vi "obsleftright.vi"(11 "update":bool=TRUE) -> ()   [LabVIEW 2015]
uses:
  G_SEN.vi
  <vilib>/Analysis/1siggen.llb/Ramp Pattern by Delta.vi
  G_ALL.vi
  <vilib>/Analysis/polynomials.llb/nth Derivative of Polynomial (DBL).vi
  <vilib>/Analysis/polynomials.llb/Scalar Polynomial Evaluation (DBL).vi
  <vilib>/Analysis/NI_AALPro.lvlib
  G_LCM.vi
  <vilib>/Analysis/NI_AALBase.lvlib
panel:
  out "x_car":dbl[](array[numeric])=[0.9, 0.9, -0.9, -0.9, 0.9]
  out "y_car":dbl[](array[numeric])=[0.0, 3.7, 3.7, 0.0, 0.0]
  out "y_ramp":dbl[](array[numeric])=[-1.0, -0.75, -0.5, -0.25, 0.0, 0.25, 0.5, 0.75, 1.0, 1.25, 1.5, 1.75, 2.0, 2.25, 2.5, 2.75, 3.0, 3.25, 3.5, 3.75, 4.0, 4.25, 4.5, 4.75, 5.0, 5.25, 5.5, 5.75, 6.0]
  out "rin":dbl[](array[numeric])=[-3.7555, -4.035824427641933, -4.343004633055794, -4.681538421297181, -5.056978730736188, -5.476262963548993, -5.94817384988562, -6.483997508991062, -7.098484710034956, -7.811291873800975, -8.649206492141174, -9.649704845388673, -10.866875707952016, -12.381774570932784, -14.321624936294773, -16.89815033646731, -20.49170207506112, -25.860884248621495, -34.76835875277913, -52.46351887551581, -104.73868975677755, -4879.314687241169, 109.5221450101935, 53.65969083607183, 35.30050875601431, 26.160648564205243, 20.683909481852254, 17.031933528233147, 14.42018130844496, 12.457468347457555, 10.92689587838567, 9.698514680927435, 8.689722854776836, 7.845501286784753, 7.127786761742499, 6.509406661367354, 5.970443364939505, 5.495963884688509, 5.074551847557845, 4.697329415527146, 4.357288430183145, 4.048822433014104, 3.767392532060661]
  out "rout":dbl[](array[numeric])=[-6.67484683344869, -6.909909315632319, -7.171227643977352, -7.463266061634917, -7.791543962127691, -8.162965313825287, -8.586279637191614, -9.072740199574223, -9.637065431692674, -10.298880108215295, -11.084940970316678, -12.032694671041764, -13.196201733859061, -14.656491052798271, -16.540761487505993, -19.06071420501164, -22.596680760750772, -27.907248474466925, -36.75506579877062, -54.389516276148846, -106.60291935538585, -4881.116089584579, 111.38361625333661, 55.58297677916027, 37.28455108962819, 28.204394482615516, 22.786315752840025, 19.19197020662005, 16.636835086002, 14.729745540190233, 13.253825059177073, 12.079148971161162, 11.1231418929198, 10.330812895090412, 9.66412833436853, 9.095946298432954, 8.60638077752387, 8.180531095636704, 7.807013712346161, 7.476983986466357, 7.183467186008942, 6.920890394517821, 6.684748282923211]
  out "r":dbl[](array[numeric])=[-4.6555, -4.935824427641934, -5.2430046330557945, -5.581538421297181, -5.956978730736188, -6.376262963548993, -6.848173849885621, -7.3839975089910626, -7.9984847100349565, -8.711291873800976, -9.549206492141174, -10.549704845388673, -11.766875707952016, -13.281774570932784, -15.221624936294774, -17.79815033646731, -21.39170207506112, -26.760884248621494, -35.66835875277913, -53.36351887551581, -105.63868975677755, -4880.214687241169, 110.4221450101935, 54.55969083607183, 36.20050875601431, 27.06064856420524, 21.583909481852253, 17.931933528233145, 15.32018130844496, 13.357468347457555, 11.82689587838567, 10.598514680927435, 9.589722854776836, 8.745501286784753, 8.0277867617425, 7.409406661367354, 6.870443364939505, 6.395963884688509, 5.974551847557845, 5.597329415527146, 5.257288430183145, 4.948822433014104, 4.667392532060661]
  out "theta":dbl[](array[numeric])=[-3.141592653589793, -3.1315926535897933, -3.121592653589793, -3.1115926535897933, -3.101592653589793, -3.0915926535897933, -3.081592653589793, -3.0715926535897933, -3.061592653589793, -3.0515926535897933, -3.041592653589793, -3.0315926535897932, -3.021592653589793, -3.0115926535897932, -3.001592653589793, -2.991592653589793, -2.981592653589793, -2.971592653589793, -2.961592653589793, -2.951592653589793, -2.941592653589793, -2.931592653589793, -2.921592653589793, -2.911592653589793, -2.901592653589793, -2.891592653589793, -2.8815926535897933, -2.871592653589793, -2.861592653589793, -2.851592653589793, -2.8415926535897933, -2.831592653589793, -2.8215926535897933, -2.811592653589793, -2.8015926535897933, -2.791592653589793, -2.7815926535897932, -2.771592653589793, -2.7615926535897932, -2.751592653589793, -2.741592653589793, -2.731592653589793, -2.721592653589793, -2.711592653589793, -2.701592653589793, -2.691592653589793, -2.681592653589793, -2.671592653589793, -2.661592653589793, -2.651592653589793, -2.641592653589793, -2.6315926535897933, -2.621592653589793, -2.611592653589793, -2.601592653589793, -2.5915926535897933, -2.581592653589793, -2.571592653589793, -2.561592653589793, -2.5515926535897933, -2.541592653589793, -2.5315926535897932, -2.521592653589793, -2.5115926535897932, -2.501592653589793, -2.491592653589793, -2.481592653589793, -2.471592653589793, -2.461592653589793, -2.451592653589793, -2.441592653589793, -2.431592653589793, -2.4215926535897934, -2.411592653589793, -2.401592653589793, -2.391592653589793, -2.3815926535897933, -2.371592653589793, -2.361592653589793, -2.351592653589793, -2.3415926535897933, -2.331592653589793, -2.321592653589793, -2.311592653589793, -2.3015926535897933, -2.291592653589793, -2.2815926535897932, -2.271592653589793, -2.2615926535897932, -2.251592653589793, -2.241592653589793, -2.231592653589793, -2.221592653589793, -2.211592653589793, -2.201592653589793, -2.191592653589793, -2.181592653589793, -2.1715926535897934, -2.161592653589793, -2.151592653589793, -2.141592653589793, -2.1315926535897933, -2.121592653589793, -2.111592653589793, -2.101592653589793, -2.0915926535897933, -2.081592653589793, -2.071592653589793, -2.061592653589793, -2.0515926535897933, -2.041592653589793, -2.031592653589793, -2.021592653589793, -2.0115926535897932, -2.001592653589793, -1.991592653589793, -1.9815926535897932, -1.9715926535897932, -1.9615926535897932, -1.9515926535897932, -1.9415926535897932, -1.9315926535897932, -1.9215926535897931, -1.9115926535897931, -1.9015926535897931, -1.8915926535897931, -1.881592653589793, -1.871592653589793, -1.861592653589793, -1.851592653589793, -1.841592653589793, -1.831592653589793, -1.821592653589793, -1.811592653589793, -1.801592653589793, -1.791592653589793, -1.781592653589793, -1.771592653589793, -1.761592653589793, -1.751592653589793, -1.741592653589793, -1.7315926535897932, -1.7215926535897932, -1.7115926535897932, -1.7015926535897932, -1.6915926535897932, -1.6815926535897932, -1.6715926535897931, -1.6615926535897931, -1.6515926535897931, -1.6415926535897931, -1.631592653589793, -1.621592653589793, -1.611592653589793, -1.601592653589793, -1.591592653589793, -1.581592653589793, -1.571592653589793, -1.561592653589793, -1.551592653589793, -1.541592653589793, -1.531592653589793, -1.521592653589793, -1.511592653589793, -1.501592653589793, -1.491592653589793, -1.481592653589793, -1.4715926535897932, -1.4615926535897932, -1.4515926535897932, -1.4415926535897932, -1.4315926535897932, -1.4215926535897931, -1.4115926535897931, -1.4015926535897931, -1.3915926535897931, -1.381592653589793, -1.371592653589793, -1.361592653589793, -1.351592653589793, -1.341592653589793, -1.331592653589793, -1.321592653589793, -1.311592653589793, -1.301592653589793, -1.291592653589793, -1.281592653589793, -1.271592653589793, -1.261592653589793, -1.251592653589793, -1.241592653589793, -1.231592653589793, -1.2215926535897932, -1.2115926535897932, -1.2015926535897932, -1.1915926535897932, -1.1815926535897932, -1.1715926535897931, -1.1615926535897931, -1.1515926535897931, -1.1415926535897931, -1.1315926535897929, -1.121592653589793, -1.1115926535897929, -1.101592653589793, -1.0915926535897933, -1.081592653589793, -1.0715926535897933, -1.061592653589793, -1.0515926535897933, -1.041592653589793, -1.0315926535897932, -1.021592653589793, -1.0115926535897932, -1.001592653589793, -0.9915926535897932, -0.981592653589793, -0.9715926535897932, -0.961592653589793, -0.9515926535897932, -0.9415926535897929, -0.9315926535897932, -0.9215926535897929, -0.9115926535897931, -0.9015926535897929, -0.8915926535897931, -0.8815926535897929, -0.8715926535897931, -0.8615926535897929, -0.8515926535897931, -0.8415926535897928, -0.8315926535897931, -0.8215926535897933, -0.811592653589793, -0.8015926535897933, -0.791592653589793, -0.7815926535897932, -0.771592653589793, -0.7615926535897932, -0.751592653589793, -0.7415926535897932, -0.731592653589793, -0.7215926535897932, -0.711592653589793, -0.7015926535897932, -0.6915926535897929, -0.6815926535897932, -0.6715926535897929, -0.6615926535897931, -0.6515926535897929, -0.6415926535897931, -0.6315926535897929, -0.6215926535897931, -0.6115926535897929, -0.6015926535897931, -0.5915926535897928, -0.5815926535897931, -0.5715926535897933, -0.561592653589793, -0.5515926535897933, -0.541592653589793, -0.5315926535897932, -0.521592653589793, -0.5115926535897932, -0.501592653589793, -0.4915926535897932, -0.481592653589793, -0.4715926535897932, -0.46159265358979296, -0.45159265358979317, -0.44159265358979294, -0.43159265358979315, -0.4215926535897929, -0.41159265358979313, -0.4015926535897929, -0.3915926535897931, -0.3815926535897929, -0.3715926535897931, -0.36159265358979287, -0.3515926535897931, -0.34159265358979285, -0.33159265358979306, -0.3215926535897933, -0.31159265358979304, -0.30159265358979326, -0.291592653589793, -0.28159265358979324, -0.271592653589793, -0.2615926535897932, -0.251592653589793, -0.2415926535897932, -0.23159265358979297, -0.2215926535897932, -0.21159265358979296, -0.20159265358979317, -0.19159265358979294, -0.18159265358979315, -0.17159265358979292, -0.16159265358979313, -0.1515926535897929, -0.14159265358979312, -0.13159265358979289, -0.1215926535897931, -0.11159265358979287, -0.10159265358979308, -0.09159265358979285, -0.08159265358979306, -0.07159265358979283, -0.061592653589793045, -0.05159265358979326, -0.04159265358979303, -0.03159265358979324, -0.02159265358979301, -0.011592653589793223, -0.0015926535897929917, 0.008407346410206795, 0.018407346410207026, 0.028407346410206813, 0.038407346410207044, 0.04840734641020683, 0.05840734641020706, 0.06840734641020685, 0.07840734641020708, 0.08840734641020687, 0.0984073464102071, 0.10840734641020688, 0.11840734641020711, 0.1284073464102069, 0.13840734641020713, 0.14840734641020692, 0.15840734641020715, 0.16840734641020694, 0.17840734641020717, 0.18840734641020696, 0.19840734641020674, 0.20840734641020697, 0.21840734641020676, 0.228407346410207, 0.23840734641020678, 0.248407346410207, 0.2584073464102068, 0.268407346410207, 0.2784073464102068, 0.28840734641020704, 0.29840734641020683, 0.30840734641020706, 0.31840734641020685, 0.3284073464102071, 0.33840734641020687, 0.3484073464102071, 0.3584073464102069, 0.3684073464102071, 0.3784073464102069, 0.38840734641020713, 0.3984073464102069, 0.40840734641020715, 0.41840734641020694, 0.42840734641020717, 0.43840734641020696, 0.44840734641020674, 0.458407346410207, 0.46840734641020676, 0.478407346410207, 0.4884073464102068, 0.498407346410207, 0.5084073464102068, 0.518407346410207, 0.5284073464102068, 0.538407346410207, 0.5484073464102068, 0.5584073464102071, 0.5684073464102068, 0.5784073464102071, 0.5884073464102069, 0.5984073464102071, 0.6084073464102069, 0.6184073464102071, 0.6284073464102069, 0.6384073464102071, 0.6484073464102069, 0.6584073464102072, 0.6684073464102069, 0.6784073464102072, 0.688407346410207, 0.6984073464102067, 0.708407346410207, 0.7184073464102068, 0.728407346410207, 0.7384073464102068, 0.748407346410207, 0.7584073464102068, 0.768407346410207, 0.7784073464102068, 0.788407346410207, 0.7984073464102068, 0.8084073464102071, 0.8184073464102068, 0.8284073464102071, 0.8384073464102069, 0.8484073464102071, 0.8584073464102069, 0.8684073464102067, 0.8784073464102073, 0.8884073464102071, 0.8984073464102069, 0.9084073464102067, 0.9184073464102074, 0.9284073464102072, 0.938407346410207, 0.9484073464102067, 0.9584073464102065, 0.9684073464102072, 0.978407346410207, 0.9884073464102068, 0.9984073464102066, 1.0084073464102072, 1.018407346410207, 1.0284073464102068, 1.0384073464102066, 1.0484073464102073, 1.058407346410207, 1.0684073464102068, 1.0784073464102066, 1.0884073464102073, 1.098407346410207, 1.1084073464102069, 1.1184073464102067, 1.1284073464102073, 1.1384073464102071, 1.148407346410207, 1.1584073464102067, 1.1684073464102074, 1.1784073464102072, 1.188407346410207, 1.1984073464102067, 1.2084073464102074, 1.2184073464102072, 1.228407346410207, 1.2384073464102068, 1.2484073464102066, 1.2584073464102072, 1.268407346410207, 1.2784073464102068, 1.2884073464102066, 1.2984073464102073, 1.308407346410207, 1.3184073464102068, 1.3284073464102066, 1.3384073464102073, 1.348407346410207, 1.3584073464102069, 1.3684073464102067, 1.3784073464102073, 1.3884073464102071, 1.398407346410207, 1.4084073464102067, 1.4184073464102074, 1.4284073464102072, 1.438407346410207, 1.4484073464102067, 1.4584073464102074, 1.4684073464102072, 1.478407346410207, 1.4884073464102068, 1.4984073464102066, 1.5084073464102072, 1.518407346410207, 1.5284073464102068, 1.5384073464102066, 1.5484073464102073, 1.558407346410207, 1.5684073464102068, 1.5784073464102066, 1.5884073464102073, 1.598407346410207, 1.6084073464102069, 1.6184073464102067, 1.6284073464102073, 1.6384073464102071, 1.648407346410207, 1.6584073464102067, 1.6684073464102074, 1.6784073464102072, 1.688407346410207, 1.6984073464102067, 1.7084073464102074, 1.7184073464102072, 1.728407346410207, 1.7384073464102068, 1.7484073464102066, 1.7584073464102072, 1.768407346410207, 1.7784073464102068, 1.7884073464102066, 1.7984073464102073, 1.808407346410207, 1.8184073464102068, 1.8284073464102066, 1.8384073464102073, 1.848407346410207, 1.8584073464102069, 1.8684073464102067, 1.8784073464102073, 1.8884073464102071, 1.898407346410207, 1.9084073464102067, 1.9184073464102074, 1.9284073464102072, 1.938407346410207, 1.9484073464102067, 1.9584073464102074, 1.9684073464102072, 1.978407346410207, 1.9884073464102068, 1.9984073464102066, 2.0084073464102072, 2.018407346410207, 2.028407346410207, 2.0384073464102066, 2.0484073464102073, 2.058407346410207, 2.068407346410207, 2.0784073464102066, 2.0884073464102073, 2.098407346410207, 2.108407346410207, 2.1184073464102067, 2.1284073464102073, 2.138407346410207, 2.148407346410207, 2.1584073464102067, 2.1684073464102074, 2.178407346410207, 2.188407346410207, 2.1984073464102067, 2.2084073464102074, 2.218407346410207, 2.228407346410207, 2.2384073464102068, 2.2484073464102066, 2.2584073464102072, 2.268407346410207, 2.278407346410207, 2.2884073464102066, 2.2984073464102073, 2.308407346410207, 2.318407346410207, 2.3284073464102066, 2.3384073464102073, 2.348407346410207, 2.358407346410207, 2.3684073464102067, 2.3784073464102073, 2.388407346410207, 2.398407346410207, 2.4084073464102067, 2.4184073464102074, 2.428407346410207, 2.438407346410207, 2.4484073464102067, 2.4584073464102074, 2.468407346410207, 2.478407346410207, 2.4884073464102068, 2.4984073464102066, 2.5084073464102072, 2.518407346410207, 2.528407346410207, 2.5384073464102066, 2.5484073464102073, 2.558407346410207, 2.568407346410207, 2.5784073464102066, 2.5884073464102073, 2.598407346410207, 2.608407346410207, 2.6184073464102067, 2.6284073464102073, 2.638407346410207, 2.648407346410207, 2.6584073464102067, 2.6684073464102074, 2.678407346410207, 2.688407346410207, 2.6984073464102067, 2.7084073464102074, 2.718407346410207, 2.728407346410207, 2.7384073464102068, 2.7484073464102066, 2.7584073464102072, 2.768407346410207, 2.778407346410207, 2.7884073464102066, 2.7984073464102073, 2.808407346410207, 2.818407346410207, 2.8284073464102066, 2.8384073464102073, 2.848407346410207, 2.858407346410207, 2.8684073464102067, 2.8784073464102073, 2.888407346410207, 2.898407346410207, 2.9084073464102067, 2.9184073464102074, 2.928407346410207, 2.938407346410207, 2.9484073464102067, 2.9584073464102074, 2.968407346410207, 2.978407346410207, 2.9884073464102068, 2.9984073464102075, 3.0084073464102072, 3.018407346410207, 3.028407346410207, 3.0384073464102066, 3.0484073464102073, 3.058407346410207, 3.068407346410207, 3.0784073464102066, 3.0884073464102073, 3.098407346410207, 3.108407346410207, 3.1184073464102067, 3.1284073464102073, 3.138407346410207, -3.141592653589793]
  out "gap":dbl=0.9
  out "af":dbl=3.7
  out "XY Graph":cluster{"Y":dbl[], "Y":dbl[]}[](graph)=[{"Y"=array[586 elements], "Y"=array[586 elements]}, {"Y"=[], "Y"=[]}, {"Y"=[], "Y"=[]}, {"Y"=array[630 elements], "Y"=array[630 elements]}, {"Y"=array[630 elements], "Y"=array[630 elements]}, {"Y"=array[630 elements], "Y"=array[630 elements]}, {"Y"=[7.816394639851724, 7.319850750911751, 6.817348511778361, 6.318251688313182, 5.827348177464875, 5.357007078148591, 4.915309928811384, 4.506393003662533, 4.139164703638908, 3.8204251317486726, 3.553125525255061, 3.3414092817759076, 3.162481577170565, 2.974816018164504, 2.7663181983145737, 2.5568038965593267, 2.346281212841328, 2.137110915736132, 1.9078677144083886, 1.6966257339926898, 1.4727897553614842, 1.267204576151037, 1.056195582801043, 0.8646221231359237, 0.6899396920978118, 0.5334627663349991, 0.38672572067820976, 0.24339724215034841, 0.1456482869244913, 0.07690190270719764, 0.07504130918645387, 0.15056146198230025, 0.2713581716204574, 0.48389367093431557, 0.7635759918697156, 1.093879975509565, 1.4677637527600913, 1.8763550195382899, 2.3153426039393317, 2.771874137881789, 3.231370665823273, 3.6509816858036017, 4.070592705783319, 4.490203725763379, 4.909814747693659, 5.329425767673296, 5.749036787653171, 6.221881697921817, 6.699225266787154, 7.177159239828125, 7.6557860912435425, 8.133025174001979, 8.628550403441674, 9.124008743619601, 9.613616845908991, 10.086525367124885, 10.584289234819206, 11.080641638604668, 11.582849558630004, 12.062121491179392, 12.540326896884341, 13.046909151428244, 13.554940980687112, 14.041806127624989, 14.542723876848166, 15.020985202042274, 15.505141607780933, 15.99311310838169, 16.493060444282225, 16.97550279588125, 17.462933231924865, 17.955771199982937, 18.449162785063116, 18.938182613989092, 19.427658560604403, 19.922519917978587, 20.42188019851678, 20.931285131759044, 21.43952238396465, 21.956510957892004, 22.463501299867655], "Y"=[-11.502422251196494, -11.568849855643048, -11.569869129213243, -11.520860138841421, -11.405170845617462, -11.226259490137743, -10.988893406280077, -10.696478505477039, -10.350566631066288, -9.958991100165163, -9.530708293774902, -9.076698909741534, -8.606503294262685, -8.139646975484823, -7.675177371218184, -7.212748738665048, -6.758736023816151, -6.300936320923626, -5.855089012523531, -5.394632350417117, -4.92904856027104, -4.473226890410778, -4.019265331616374, -3.5554085848815493, -3.086532078701303, -2.6094805590208754, -2.1284651391769147, -1.6493875550133497, -1.154198294196969, -0.6553479932436498, -0.14705148394533343, 0.3495082078877353, 0.840275199270352, 1.2950552074773085, 1.7139922024325969, 2.091455354026735, 2.424471695783147, 2.7142412798840154, 2.9593516326772193, 3.1677381667356266, 3.373124974874619, 3.571397041456308, 3.76966910803638, 3.9679411746171946, 4.166213251006239, 4.364485317587152, 4.562757384167902, 4.728902132967184, 4.893725317609852, 5.06325165554511, 5.223036909273246, 5.382011198665163, 5.546222380223215, 5.708907308255361, 5.868935992202126, 6.031944130466162, 6.194471477185138, 6.35598661708894, 6.520343533121731, 6.686404463094906, 6.851993294039719, 7.0204856344182245, 7.184294420682817, 7.35241936258849, 7.5192717503812485, 7.678685140450257, 7.845257459374583, 8.007859664044247, 8.172687410639393, 8.329345654397303, 8.483897842226659, 8.635186977264295, 8.778973143211905, 8.910395437670521, 9.02767533114414, 9.127472540585499, 9.208969224478702, 9.27032570434919, 9.307930968543975, 9.319536747877331, 9.309462952310396]}, {"Y"=[-0.8366356389407819, -0.25840338682322134, 0.16096387556169744, 1.0225238690494292, 1.789749584208254, 2.5228442391661003, 3.2582102778678763, 3.9651965467946226, 4.668134133038354, 5.307553335275859, 5.78252262984093, 6.192213941390776, 6.6118249613773, 7.031435981354307, 7.451046959879165, 7.870658023263255, 8.29026904324418, 8.941462638036167, 9.425515144535234, 9.885483743848654, 10.401757606348562, 10.881711564834836, 11.36208862651888, 11.863127252302835, 12.361307835200675, 12.818353134972247, 13.324432307326454, 13.824206750930301, 14.31718322119306, 14.784287511760091, 15.263954206446822, 15.767174370388378, 16.292185876084783, 16.75852144103834, 17.267766359662545, 17.768273946512444, 18.22690912729219, 18.730869971236952, 19.225262001281948, 19.734216994347804, 20.230432724257977, 20.735913809073367, 21.2561960050937, 21.788791728779202, 22.326632476864347], "Y"=[3.041332836906522, 3.6462076206641867, 4.157380552096733, 4.573336958069159, 4.872028835248066, 5.091117493868304, 5.224453014781301, 5.298985470194547, 5.303829930891121, 5.314489619988054, 5.499260342882392, 5.767578377538095, 5.965850444112123, 6.164122510695547, 6.362394628537478, 6.560666653667127, 6.758938720246449, 6.638430091943965, 6.7872346473437695, 6.978852871826557, 7.088582585204193, 7.246253367993072, 7.400215653030386, 7.555578647491765, 7.71387478720567, 7.925551006627789, 8.035929820683164, 8.195204964883214, 8.362176683901211, 8.582089160559374, 8.747536982716873, 8.873738921644886, 9.01251449475196, 9.242709401695103, 9.375580399508735, 9.543086650041982, 9.733448334959586, 9.868788167121654, 10.021119094451475, 10.171413059138207, 10.30556202953376, 10.430073101962705, 10.534448967040744, 10.608420742432445, 10.647751914269572]}, {"Y"=[7.935733401581995, 7.3216763036249155, 6.729395708788731, 6.11180757566516, 5.507368188988451, 4.930972520387127, 4.391802788109021, 3.8892949913512833, 3.4411722551162045, 3.0569246353311437, 2.7374541534178105, 2.500254660428585, 2.3274230818952644, 2.1537473135747893, 1.946534501105246, 1.740311192177928, 1.5276801193422518, 1.3367156085885759, 1.0898435638455792, 0.885496931363002, 0.6523741827186508, 0.45106216037155633, 0.22434793239093076, 0.02124995471198088, -0.16523154823900843, -0.32737353443336026, -0.47551325407460976, -0.6395645619386285, -0.7459253719982921, -0.8230920678538325, -0.8147271750975142, -0.7233550174119514, -0.5439971002335124, -0.26462901118463134, 0.08627806496138235, 0.49527482617146334, 0.9471285592689194, 1.4375971487852823, 1.9416240656384702, 2.404609064220973, 2.8468708880536386, 3.2664819080360727, 3.6860929280148693, 4.105703933906775, 4.525314969924736, 4.94492598990481, 5.45068332709565, 5.928136581982702, 6.39835592960634, 6.892164252318939, 7.371350837869192, 7.849916247346979, 8.347781498446727, 8.844399816673128, 9.320327769778217, 9.807175868720792, 10.30579893647544, 10.800709622012374, 11.288197958814006, 11.767632746974252, 12.256280932305932, 12.770717292259999, 13.261173965936324, 13.7573855438323, 14.258130217576293, 14.72818774974823, 15.22062317451208, 15.711312191139838, 16.21510047159616, 16.703481603659235, 17.198819483826192, 17.703964418340465, 18.21557926361523, 18.72847553273765, 19.249740131820566, 19.777555829433023, 20.314255449157223, 20.86487427625775, 21.41932354206416, 21.974390246783386, 22.481380588759038], "Y"=[-12.394475085925853, -12.468848004172973, -12.46556121048128, -12.396862894746317, -12.246368091793784, -12.019035975405181, -11.720972823852813, -11.351604480539473, -10.9187272965521, -10.435506568927917, -9.911076816611818, -9.396790932425702, -8.94217770417287, -8.508220146433779, -8.046599893138712, -7.591350988647731, -7.132757747412678, -6.712478970349138, -6.230370892043438, -5.78459397102167, -5.299073273182397, -4.852583658065757, -4.362819528952363, -3.8696113626030337, -3.3670354649567713, -2.872084563711297, -2.3864262804699528, -1.8236817101647458, -1.2770657460100523, -0.6586423753999348, -0.011729481392127039, 0.5646128034759201, 1.2213208404472837, 1.7947689198701726, 2.3066704610229336, 2.7635207341691057, 3.1585963413975073, 3.5000475733509786, 3.7780911847511787, 3.989392817832373, 4.186857068929599, 4.385129135512282, 4.583401202091919, 4.781673262015884, 4.979945345061554, 5.178217411642675, 5.411865865207488, 5.579615837371853, 5.741945596749875, 5.916936525444208, 6.076908437454078, 6.236323399004274, 6.401306482512538, 6.564371420870169, 6.719807026979052, 6.887492993910782, 7.050300405025509, 7.21134506013289, 7.370743694649158, 7.536861034317964, 7.705994400600314, 7.877059073726956, 8.035000563275199, 8.2062957772499, 8.37309049525761, 8.529725475528517, 8.699101274794145, 8.862604212457192, 9.028688726984386, 9.187252683732133, 9.344272137557052, 9.499243309177244, 9.648132932035574, 9.785622802458096, 9.90991397952625, 10.015721049186642, 10.102511004881439, 10.167872136725581, 10.20770427709779, 10.219359136478959, 10.209285340912023]}, {"Y"=[0.9633523021812784, 1.521133581744715, 1.9087968343502006, 2.653234412757369, 3.286794948446148, 3.8774400929827664, 4.455420576544079, 5.0064669337769665, 5.5456498745443685, 6.054990411877582, 6.5170527771625615, 6.9612134969300445, 7.380824516912359, 7.800435536891207, 8.220046543592373, 8.639657578801101, 9.05926859878115, 9.53816955915121, 10.013005376413464, 10.487222418210283, 10.971747581366934, 11.450582071583536, 11.92830647982888, 12.424665062292728, 12.92052568909362, 13.404931287233795, 13.88313130413464, 14.381187347617834, 14.877047254377649, 15.373590711392088, 15.852931694857102, 16.335266299545196, 16.844569594421273, 17.346055470539916, 17.836607527247924, 18.33746126505619, 18.812504031880277, 19.299906837774657, 19.788863835765653, 20.290136939719932, 20.774475108702013, 21.26414130527071, 21.759809568378643, 22.255958771674976, 22.746046639367226], "Y"=[3.0479216012190924, 3.3755636155577737, 3.727171360920363, 3.8112456757152957, 3.8726014104623374, 3.9057609766876302, 3.8803222544965603, 3.830736178965827, 3.732217343957194, 3.6770105158401343, 3.8559510406889004, 4.140114189428136, 4.338386256000174, 4.5366583225844686, 4.734930453740099, 4.933202465556496, 5.131474532135405, 4.940213129864795, 5.08580723853443, 5.282412313546512, 5.381212845405997, 5.538510311631407, 5.691591252352165, 5.845410442913117, 6.002946561976053, 6.223808937073938, 6.324832093793923, 6.483547109202469, 6.65145979781331, 6.881288837504521, 7.046623840270758, 7.1657367085236965, 7.2993676161344965, 7.541297116510339, 7.667827570185912, 7.835449160289259, 8.031367664803067, 8.161100536282527, 8.311629997625584, 8.459410426448219, 8.589747970864101, 8.709324511301917, 8.806336303214847, 8.870101164785106, 8.897297184694423]}, {"Y"=[7.6970558781214535, 7.318025198198587, 6.905301314767991, 6.5246958009612035, 6.1473281659413, 5.783041635910055, 5.438817069513747, 5.123491015973782, 4.837157152161612, 4.5839256281662015, 4.368796897092311, 4.1825639031232305, 3.997540072445866, 3.7958847227542183, 3.5861018955239015, 3.3732966009407255, 3.164882306340404, 2.9375062228836883, 2.725891864971198, 2.5077545366223775, 2.2932053280043174, 2.083346991930518, 1.8880432332111552, 1.7079942915598665, 1.545110932434632, 1.3942990671033586, 1.2489646954310292, 1.1263590462393254, 1.0372219458472747, 0.9768958732682278, 0.9648097934704221, 1.024477941376552, 1.0867134434744272, 1.2324163530532624, 1.4408739187780488, 1.6924851248476664, 1.9883989462512632, 2.3151128902912976, 2.689061142240193, 3.139139211542605, 3.6158704435929074, 4.035481463571131, 4.45509248355177, 4.8747035176199836, 5.294314525462582, 5.713925545441782, 6.047390248210693, 6.515626813860932, 7.000094603967969, 7.462154227337311, 7.940221344617893, 8.41613410065698, 8.90931930843662, 9.403617670566074, 9.906905922039765, 10.365874865528978, 10.862779533162971, 11.360573655196962, 11.877501158446002, 12.356610235384531, 12.82437286146275, 13.323101010596488, 13.8487079954379, 14.326226711417679, 14.82731753612004, 15.313782654336318, 15.789660041049787, 16.27491402562354, 16.77102041696829, 17.247523988103268, 17.727046980023538, 18.20757798162541, 18.682746306511003, 19.147889695240533, 19.60557698938824, 20.06748400652415, 20.52950494787634, 20.997695987260336, 21.45972122586514, 21.93863166900062, 22.445622010976273], "Y"=[-10.610369416467135, -10.668851707113124, -10.674177047945207, -10.644857382936525, -10.563973599441141, -10.433483004870304, -10.256813988707341, -10.041352530414605, -9.782405965580475, -9.482475631402409, -9.150339770937986, -8.756606887057366, -8.2708288843525, -7.771073804535867, -7.303754849297656, -6.834146488682364, -6.384714300219623, -5.889393671498115, -5.479807133003624, -5.004670729812564, -4.559023847359684, -4.0938701227558, -3.675711134280385, -3.241205807160065, -2.8060286924458344, -2.346876554330454, -1.8705039978838767, -1.4750933998619535, -1.0313308423838858, -0.6520536110873648, -0.2823734864985398, 0.13440361229955045, 0.45922955809342025, 0.7953414950844444, 1.1213139438422601, 1.4193899738843643, 1.690347050168787, 1.9284349864170522, 2.14061208060326, 2.34608351563888, 2.55939288081964, 2.7576649474003334, 2.955937013980841, 3.154209087218505, 3.3524811569509234, 3.55075322353163, 3.713648903128317, 3.8781884285625137, 4.0455050384698295, 4.209566785646012, 4.369165381092413, 4.527698998326052, 4.6911382779338915, 4.853443195640552, 5.0180649574252, 5.176395267021541, 5.338642549344766, 5.500628174044989, 5.669943371594305, 5.835947891871848, 5.997992187479124, 6.163912195109493, 6.333588278090435, 6.4985429479270795, 6.6654530055048875, 6.827644805371998, 6.99141364395502, 7.1531151156313015, 7.316686094294399, 7.471438625062473, 7.623523546896266, 7.771130645351347, 7.909813354388237, 8.035168072882946, 8.14543668276203, 8.239224031984357, 8.315427444075965, 8.3727792719728, 8.40815765999016, 8.419714359275703, 8.409640563708768]}, {"Y"=[0.9, 0.9, -0.9, -0.9, 0.9], "Y"=[0.0, 3.7, 3.7, 0.0, 0.0]}, {"Y"=[7.816394639851724, 7.319850750911751, 6.817348511778361, 6.318251688313182, 5.827348177464875, 5.357007078148591, 4.915309928811384, 4.506393003662533, 4.139164703638908, 3.8204251317486726, 3.553125525255061, 3.3414092817759076, 3.162481577170565, 2.974816018164504, 2.7663181983145737, 2.5568038965593267, 2.346281212841328, 2.137110915736132, 1.9078677144083886, 1.6966257339926898, 1.4727897553614842, 1.267204576151037, 1.056195582801043, 0.8646221231359237, 0.6899396920978118, 0.5334627663349991, 0.38672572067820976, 0.24339724215034841, 0.1456482869244913, 0.07690190270719764, 0.07504130918645387, 0.15056146198230025, 0.2713581716204574, 0.48389367093431557, 0.7635759918697156, 1.093879975509565, 1.4677637527600913, 1.8763550195382899, 2.3153426039393317, 2.771874137881789, 3.231370665823273, 3.6509816858036017, 4.070592705783319, 4.490203725763379, 4.909814747693659, 5.329425767673296, 5.749036787653171, 6.221881697921817, 6.699225266787154, 7.177159239828125, 7.6557860912435425, 8.133025174001979, 8.628550403441674, 9.124008743619601, 9.613616845908991, 10.086525367124885, 10.584289234819206, 11.080641638604668, 11.582849558630004, 12.062121491179392, 12.540326896884341, 13.046909151428244, 13.554940980687112, 14.041806127624989, 14.542723876848166, 15.020985202042274, 15.505141607780933, 15.99311310838169, 16.493060444282225, 16.97550279588125, 17.462933231924865, 17.955771199982937, 18.449162785063116, 18.938182613989092, 19.427658560604403, 19.922519917978587, 20.42188019851678, 20.931285131759044, 21.43952238396465, 21.956510957892004, 22.463501299867655], "Y"=[-11.502422251196494, -11.568849855643048, -11.569869129213243, -11.520860138841421, -11.405170845617462, -11.226259490137743, -10.988893406280077, -10.696478505477039, -10.350566631066288, -9.958991100165163, -9.530708293774902, -9.076698909741534, -8.606503294262685, -8.139646975484823, -7.675177371218184, -7.212748738665048, -6.758736023816151, -6.300936320923626, -5.855089012523531, -5.394632350417117, -4.92904856027104, -4.473226890410778, -4.019265331616374, -3.5554085848815493, -3.086532078701303, -2.6094805590208754, -2.1284651391769147, -1.6493875550133497, -1.154198294196969, -0.6553479932436498, -0.14705148394533343, 0.3495082078877353, 0.840275199270352, 1.2950552074773085, 1.7139922024325969, 2.091455354026735, 2.424471695783147, 2.7142412798840154, 2.9593516326772193, 3.1677381667356266, 3.373124974874619, 3.571397041456308, 3.76966910803638, 3.9679411746171946, 4.166213251006239, 4.364485317587152, 4.562757384167902, 4.728902132967184, 4.893725317609852, 5.06325165554511, 5.223036909273246, 5.382011198665163, 5.546222380223215, 5.708907308255361, 5.868935992202126, 6.031944130466162, 6.194471477185138, 6.35598661708894, 6.520343533121731, 6.686404463094906, 6.851993294039719, 7.0204856344182245, 7.184294420682817, 7.35241936258849, 7.5192717503812485, 7.678685140450257, 7.845257459374583, 8.007859664044247, 8.172687410639393, 8.329345654397303, 8.483897842226659, 8.635186977264295, 8.778973143211905, 8.910395437670521, 9.02767533114414, 9.127472540585499, 9.208969224478702, 9.27032570434919, 9.307930968543975, 9.319536747877331, 9.309462952310396]}]
  out "y_shift":dbl format="%#_13g"
  out "x_shift":dbl format="%#_13g"
  in  "y_gain":dbl=0.5
  out "rr_shift":dbl
  out "rf_shift":dbl
  out "lr_shift":dbl
  out "lf_shift":dbl
  in  "x_gain":dbl=0.5
  in  "x limit":dbl=0.01
  in  "d_safe":dbl=0.25
  in  "d_safe front":dbl=0.5
  in  "y limit":dbl=0.01
  out "sorted array":dbl[](array[numeric])=[3.1400636936215167, 3.157530680769389, 3.178049716414141, 3.2, 3.2, 3.2, 3.2, 3.2, 3.2, 3.2, 3.2, 3.2, 3.2, 3.2, 3.2, 3.2, 3.2, 3.2, 3.2, 3.2, 3.2, 3.2, 3.2, 3.2, 3.2, 3.2, 3.2, 3.2, 3.2, 3.2015621187164247, 3.2015621187164247, 3.2015621187164247, 3.2015621187164247, 3.2015621187164247, 3.2015621187164247, 3.2015621187164247, 3.2062439083762797, 3.2062439083762797, 3.2062439083762797, 3.2062439083762797, 3.2062439083762797, 3.2062439083762797, 3.2062439083762797, 3.2140317359976396, 3.2140317359976396, 3.2140317359976396, 3.2140317359976396, 3.2140317359976396, 3.2140317359976396, 3.2140317359976396, 3.22490309931942, 3.22490309931942, 3.22490309931942, 3.22490309931942, 3.23882694814033, 3.23882694814033, 3.23882694814033, 3.23882694814033, 3.2557641192199416, 3.2557641192199416, 3.2557641192199416, 3.2557641192199416, 3.2572994949804666, 3.2756678708318403, 3.2756678708318403, 3.2756678708318403, 3.2756678708318403, 3.2893768406797057, 3.298484500494129, 3.298484500494129, 3.298484500494129, 3.298484500494129, 3.3, 3.3, 3.3, 3.3, 3.3, 3.3, 3.3, 3.3, 3.3, 3.3, 3.3, 3.3, 3.3, 3.3, 3.3, 3.3, 3.3, 3.3, 3.3, 3.3, 3.3, 3.3, 3.3, 3.3, 3.3, 3.3, 3.3, 3.3, 3.3, 3.3, 3.3000000000000003, 3.3000000000000003, 3.3000000000000003, 3.3000000000000003, 3.3000000000000003, 3.3000000000000003, 3.3000000000000003, 3.3000000000000003, 3.3000000000000003, 3.3000000000000003, 3.3000000000000003, 3.3000000000000003, 3.3000000000000003, 3.3000000000000003, 3.3000000000000003, 3.3000000000000003, 3.3000000000000003, 3.3000000000000003, 3.3000000000000003, 3.3000000000000003, 3.3000000000000003, 3.3000000000000003, 3.3000000000000003, 3.3000000000000003, 3.3000000000000003, 3.3015148038438356, 3.3015148038438356, 3.3015148038438356, 3.3015148038438356, 3.301514803843836, 3.301514803843836, 3.301514803843836, 3.3060550509633075, 3.3060550509633075, 3.306055050963308, 3.306055050963308, 3.306055050963308, 3.3060550509633084, 3.3060550509633084, 3.313608305156178, 3.313608305156178, 3.313608305156178, 3.313608305156178, 3.3136083051561784, 3.3136083051561784, 3.3136083051561784, 3.324154027718932, 3.324154027718932, 3.3241540277189325, 3.3241540277189325, 3.3241540277189325, 3.3241540277189325, 3.3241540277189325, 3.337663853655727, 3.3376638536557275, 3.3376638536557275, 3.3376638536557275, 3.3526109228480423, 3.3526109228480423, 3.3541019662496843, 3.3541019662496847, 3.3541019662496847, 3.354101966249685, 3.3734255586865998, 3.3734255586866007, 3.3734255586866007, 3.3734255586866007, 3.383784863137726, 3.3837848631377265, 3.395585369269929, 3.395585369269929, 3.3955853692699294, 3.3955853692699294, 3.4000000000000004, 3.4000000000000004, 3.4000000000000004, 3.4000000000000004, 3.4000000000000004, 3.4000000000000004, 3.4000000000000004, 3.4000000000000004, 3.4000000000000004, 3.4000000000000004, 3.4000000000000004, 3.4000000000000004, 3.4000000000000004, 3.4000000000000004, 3.4000000000000004, 3.4000000000000004, 3.4000000000000004, 3.4000000000000004, 3.4000000000000004, 3.4000000000000004, 3.4000000000000004, 3.4000000000000004, 3.4000000000000004, 3.4000000000000004, 3.4000000000000004, 3.4000000000000004, 3.4000000000000004, 3.4000000000000004, 3.4000000000000004, 3.40147027033899, 3.405877273185281, 3.4132096331752027, 3.4176014981270124, 3.417601498127013, 3.4205262752974144, 3.423448553724738, 3.4365680554879168, 3.448187929913334, 3.452535300326414, 3.471310991541957, 3.4785054261852175, 3.4928498393145966, 3.5, 3.5, 3.5, 3.5, 3.5014282800023193, 3.505709628591621, 3.5114099732158874, 3.5128336140500593, 3.5227829907617076, 3.5355339059327378, 3.5510561809129406, 3.5693136595149495, 3.5902646142032486, 3.6, 3.6, 3.6]
  out "x":dbl[](array[numeric])=[17.023623347443277, 16.143361660154127, 16.141835960078435, 16.126620436500318, 16.074105895973318, 16.039987587227966, 15.98756727407812, 15.960794387991761, 15.925712379604642, 15.838609280398552, 15.808580937163462, 15.757599675664727, 15.722652886773686, 13.240848286646317, 12.497408954434835, 12.492977151439103, 12.48563257884241, 12.478760795745522, 12.093539497538087, 6.97374919093925, 6.9696108697295855, 6.609439488644903, 6.606090407205891, -15.235815391892325, -15.240927762567464, -28.08632975065424, -28.30674578448887, -28.5406821527515, -28.7021611146982, -28.789147331793064, -28.87360174072627, -28.947519783267502, -29.02289485501451, -29.111722874742025, -29.186, -29.275721313580224, -29.3608819850102, -29.447476947054504, -29.541500001090736, -29.61894981426939, -29.705817068973662, -29.7821028725707, -29.883784509525004, -29.970875713004244, -30.059362890954937, -30.131260426705023, -30.236505053298988, -30.317161468144455, -30.411171038317445, -30.506543001250584, -30.599279677669852, -30.695360697362172, -30.77483809234166, -30.879578660395637, -30.97567794246474, 25.94128612159452, 49.06362267779398, 48.86622739672558, 48.666561772133434, 48.45621212773354, 16.977213515699226, 16.93108142568222, 47.85563898223219, 47.673252447580005, 38.965991910946485, 38.8387521990586, 47.074286212793396, 46.841684308898124, 46.66790278123901, 46.4557507357173, 46.25131111813685, 46.05451487341698, 45.83445220545603, 45.64312078864578, 45.44637922888971, 45.27161067624044, 43.31738362170412, 44.85775932833634, 44.65889635020243, 25.63324642480981, 25.521878061303774, 11.140896034491835, 11.01642590639509, 10.810949078759245, 10.62202665972505, 10.457276057364998, 10.287031883987753, 10.123714534046886, 9.988793082298388, 9.82681811633025, 9.693052366238117, 9.529407560899587, 9.418047885862505, 9.270852483456531, 9.1303426220247, 9.026414346949053, 8.903448713986322, 8.78099925784089, 8.660552091595935, 8.55389166167106, 8.425616473265055, 8.289162854151678, 8.211654314454181, 8.1111362166594, 7.998013787925614, 7.905544405721775, 7.807691183328732, 7.697398847271927, 7.628811304945332, 7.427449629583494, 7.366810076707253, 7.327305448990642, 7.272372172469991, 7.174431650100525, 7.0838597434335675, 20.474418499435018, 20.334860786905686, 20.21033940209208, 17.814446765766522, 6.488368353940801, 6.445308216068728, 6.412947731343297, 6.375151070291986, 6.358501982678217, 19.127622096053003, 19.025711840724714, 9.376241084374545, 9.253335792608455, 9.13877756807008, 9.03245149131525, 8.917616321621233, 8.819860602371474, 5.515925054408015, 5.481380606044085, 5.449289748834418, 5.427082602206767, 8.28347704176558, 8.199379528387118, 8.10330791853597, 8.006430314322694, 7.914824187648887, 7.819984410837715, 7.724370593367207, 7.624438480578692, 7.535650158745494, 7.442536864527296, 7.358040289037849, 4.5829077264707365, 4.551366968633625, 4.522076624191647, 4.493854476309252, 4.4689452093369315, 6.821195723664231, 6.740511258436382, 6.660175953438991, 6.590127604625974, 6.540041641713532, 6.491008019309094, 6.436514260336391, 6.354105168309539, 6.237953691053496, 6.123747017478916, 6.048302838454588, 5.978428577479886, 5.911940049997303, 3.663980864910126, 3.625067980286299, 3.595401763213628, 3.5707499492986905, 3.544, 3.5171825780498764, 5.528931732841728, 5.484284814561822, 5.454108227771292, 5.417857493107981, 5.3909396734130555, 5.352298796526209, 5.324746465117574, 5.299624470340419, 5.271322168691149, 5.242656328089154, 5.225430652002183, 5.196836600218225, 5.17589463207378, 5.15443239581224, 5.129819159725784, 5.10560066501671, 5.084336053305966, 5.0650772175899155, 2.691233090764774, 2.6643505696881924, 2.6374490232936805, 2.612993340326943, 2.5900989431066965, 5.503936263609503, 5.4293673224861525, 5.3306210366131435, 5.251426366895838, 5.186567417473038, 5.11341602326233, 5.047386069307932, 5.007740940783913, 4.9669518923818465, 4.9001214013038545, 4.820425909173232, 4.742641444282501, 4.678767447797834, 4.622037017862451, 4.538979086514243, 4.470203273266491, 4.409813169943418, 4.35083860325297, 4.2648781871194155, 4.199178056188407, 4.138854555243509, 4.086883974497589, 4.060481914868296, 4.027109470694315, 3.9918931314727737, 1.7152258803723732, 1.689693894210803, 1.6653492301007082, 1.6415659432917726, 1.6171833727441358, 1.5961446960327792, 4.299391476033552, 4.259443539282746, 3.7055273227011103, 4.16115381272516, 4.059835541478139, 3.536930264471189, 3.4732714162432115, 3.820791414396031, 3.743499412509257, 3.270082506623489, 3.5591080173471337, 3.4847627435843855, 3.3972108227010507, 3.3064889714921315, 3.223651609994104, 3.1338642177507117, 3.050896151059798, 2.9715404326374686, 2.898411030557212, 2.8393445466227307, 2.7728363208119498, 2.508002188173447, 2.4332087363711548, 2.3513460098913446, 2.2504803825634174, 1.9949371553415083, 1.9267657508175495, 0.8365043114023107, 0.8115820046287177, 0.7886076340085284, 0.7662439872959019, 0.7435787671582909, 0.7217517015788992, 0.7009551355628123, 1.5195859298258414, 1.4750135512595797, 1.4348896492522059, 1.38553084123299, 1.313587711963803, 1.2656306332447473, 1.219088333695744, 1.1764107664332295, 1.2037952951357227, 1.140345738110361, 1.0818064229394369, 1.0196544080790728, 0.9592602970892483, 0.9020907184590268, 0.7216581279253979, 0.6659174692462184, 0.6142096604616322, 0.5686825005358285, 0.524784769766459, 0.5512618175231158, 0.4936529233545287, 0.16535381537644983, 0.14481362964097952, 0.12334578042669897, 0.10270447874271364, 0.08220083431960545, 0.061704353523317, 0.0, -0.04468901369437388, -0.08944698885833181, -0.13484901357598889, -0.18112107400612854, -0.10523500540672273, -0.12591112136086952, -0.14664594043356782, -0.16737798618519384, -0.1887611941696008, -0.20998373077672727, -0.23096671070174926, -0.530791268215937, -0.5765656495195518, -0.6234276857299603, -0.6655422430459373, -0.7090047991352906, -0.3382311492518023, -0.35777347651897295, -0.37694296059555393, -0.39655862950184523, -0.41614936168115435, -0.43552309945189793, -0.4548537997188262, -0.4745592232351464, -0.4940378780782147, -0.5125841519410819, -0.5317391860992575, -0.5496307387572148, -0.5686525549260484, -0.5871068126057913, -0.605210975068468, -0.6232171460991719, -0.6431339317644653, -0.6618905430383968, -0.681817016903207, -1.594692936620116, -1.6379667435029897, -1.6933884361305538, -1.9448097022021993, -1.9934810796163607, -2.0452831116763366, -2.091334890547886, -1.9253010996821598, -1.990519439768116, -2.0429858521528947, -2.0817999711843727, -2.1349801189536195, -2.287699661190804, -2.3258600913788534, -2.4978535695733486, -2.9189611906662307, -2.7444676916545103, -2.75041736659742, -2.77683580211971, -2.8098472051984893, -2.8637701295931737, -2.946375185958494, -2.9966647960582606, -3.039496242297571, -3.0763222987965726, -3.1249346684484047, -3.177295724469929, -2.9999369813919894, -3.0928057528335096, -3.1381430518463604, -3.1693931278891716, -3.2153110934188773, -3.261959244230015, -3.308025975006669, -3.3507821757209912, -3.394891942650588, -3.4230976944964078, -3.459348512081021, -3.49472679880947, -3.530641038920299, -3.572189305324163, -3.6239641298498513, -3.6655541718473006, -3.7138497671253528, -3.748621311789087, -3.7717279093903247, -3.8137435036623244, -3.8494830778763243, -3.902437764214865, -3.9284758270515256, -3.9565834811722342, -4.0112367740135415, -4.085009708093644, -4.19088991028395, -1.969401099711659, -1.9852509155013858, -1.9975714891904905, -2.011481541782451, -2.029658409633429, -2.0469120583335374, -2.068573061577074, -2.092057553941999, -2.1237675577815995, -2.1391869314264227, -4.662737496447372, -4.694325593917775, -4.722883921626059, -4.754022737204567, -4.791628270526989, -4.8300892174884895, -4.871367064235195, -4.903802779663438, -4.947871931919637, -5.002854790053447, -5.049999999999998, -5.107260579287545, -5.118016852095739, -5.019561078073389, -5.292524779753642, -5.0222562040497, -5.09690806449201, -5.142336540119021, -5.17392634631777, -5.193538014280401, -5.23446898495671, -5.2819093615757335, -5.318444326343163, -5.344957765761972, -5.37458643423163, -2.632680189540276, -2.6541880390099437, -2.67570306323291, -2.6903847194545505, -2.709575085322341, -2.735668200776487, -2.7525320100698547, -2.7728489131152636, -2.7884532368754926, -2.8158165455073783, -2.8420632750979085, -2.8671714859345983, -2.893526631315049, -2.910253494510236, -2.933012564964017, -2.9521117243261155, -2.9687196340203243, -2.98774739936926, -3.0154608998726293, -3.0244622175933737, -3.0421347703349135, -3.059762968928328, -3.081162899025489, -3.101279159605836, -3.121376632637835, -3.14145478902409, -3.1654097875613147, -3.1828565530082336, -3.205504415647618, -3.2255197274695377, -3.241537275871387, -3.260156636740084, -3.8750220060704668, -3.884084368011766, -3.906559639660766, -3.9320369129606423, -3.957519478422276, -3.9769232000881622, -4.002391071539582, -4.029393770805823, -4.059484873347866, -4.081894046121038, -4.11357372536457, -4.12819934725943, -4.161463601783617, -4.17912755759189, -4.210869383382553, -4.241073875911377, -4.266560939921778, -4.290454864295, -4.3127388497325825, -4.342979903637177, -4.373243309667808, -4.397097027576179, -4.42415509901141, -4.454447571028461, -4.481511528410799, -4.50531527858387, -4.527460781816348, -4.551208758069639, -4.679088059500656, -4.702792127183196, -4.72312929618844, -4.765158516020534, -4.7888089429683705, -5.082529517619591, -5.092228338209417, -5.141548926976563, -5.1805639654385125, -5.198774501160985, -5.230837732598797, -5.262895914663113, -5.296696946436181, -5.330498674701648, -5.367814924139284, -5.403383788151835, -5.437191276825272, -5.478073475896229, -5.504789230704044, -5.543910894305052, -5.5830468805643125, -5.615051596169229, -5.645245952985573, -5.680791944868049, -5.719925310647898, -5.753660352792691, -5.785571672682606, -5.821073316144314, -5.885562769016005, -5.9065632025583295, -5.94932678899084, -6.4125011530277645, -6.4645412623391065, -6.4979588646396715, -6.5387973071864005, -6.577741064931406, -6.6316390998786545, -6.6836750771117766, -6.720681623860816, -6.765173197662791, -6.81529798059645, -6.861639000214756, -6.921195973386999, -6.967511892824987, -7.023284990457113, -7.056264507679946, -7.096783724594435, -7.390535762691558, -7.689771016604811, -7.735664762459423, -7.773771049974421, -7.835006197080767, -7.898148450204602, -7.959324230511867, -8.020464473397388, -8.077680652567082, -8.146515193091734, -8.20169363178774, -8.276299330285788, -8.323571363219648, -8.398098253245667, -8.686052581759034, -8.932439016120336, -8.996782404210185, -9.061046743927047, -9.133107101435218, -9.209035815838678, -9.286865224074571, -9.376465482322203, -9.450202042814277, -9.517921345804536, -9.60730009669766, -9.728273132437359, -9.821478705778896, -10.017558879320982, -10.09662637784014, -10.19543406965966, -10.276272392569577, -10.364941598418161, -10.461448903451693, -10.571767747764746, -10.668052452686275, -10.732361810794922, -10.914022006218294, -10.995997077536687, -11.392586114576522, -11.454030425083303, -11.557202048949506, -11.662206984761093, -11.781021712576717, -11.871707909162375, -12.004159908776138, -12.136437795776407, -12.252546442383744, -12.470398739544276, -12.548144699364094, -12.729636376238746, -12.88093395689755, -12.952027043055892, -13.130874949701859, -13.243495709061884, -13.73, -13.843868215097848, -13.931469512130034, -14.030797844518466, -14.00586651375073, -13.64763164928448, -15.098796614604499, -15.24423817688847, -15.35337306926999, -14.097746126848595, -16.061985176204683, -16.13537878876822, -16.280245300240335, -16.41872704747793]
  out "y":dbl[](array[numeric])=[0.8913733849681116, 0.45571892022938365, 0.5222631059463902, 0.39032446108712393, 0.5922919145860788, 0.6600754677309506, 0.7283743985500302, 0.7951626687078063, 0.8620127672726878, 0.9952702613803203, 1.0610027184860518, 1.1915376147054322, 1.256591712317994, 1.178507449722868, 4.378038994907885, 4.486056245378499, 4.4297152344405175, 4.537250668655037, 1.350826043310616, 1.6788421110539233, 1.621499244132747, 2.6011114346131747, 2.544584012105102, 2.765545956473856, 2.8921281551513554, 2.486964809731412, 2.378879901618132, 2.2694088701594275, 2.156265963502494, 2.0402974537738094, 1.923596241277696, 1.80609068483809, 1.688004375636904, 1.569364135563565, 1.4500000000000017, 1.3299634366323567, 1.2092239361407566, 1.0877592169781811, 0.9654486271628676, 0.8426881384392699, 0.7190373581972689, 0.5949496849733764, 0.46936990473855067, 0.34345657808866226, 0.21672849124189253, 0.08997514098839865, -0.03906331640157967, -0.16771203240241772, -0.2978535547876131, -0.4289195927028855, -0.5606697686881945, -0.6934946182978894, -0.8259658656311124, -0.9611527080699307, -1.0965864210737275, 2.167378987671688, 33.66149096686558, 33.835007843645734, 34.00631370384796, 34.17001169795842, 14.220110679034324, 14.295172838883367, 34.675531766047555, 34.85423745029037, 29.336243400230646, 29.497069141797546, 35.351740632234154, 35.49339769433365, 35.67467612194483, 35.828666858340526, 35.98719498294877, 36.15036620456786, 36.296084116539745, 36.46166836383674, 36.622663923881326, 36.79922970426204, 35.646624556050966, 37.10274622040425, 37.25941390515854, 22.969081771271767, 23.061149364951955, 12.004221938154156, 11.98464992091835, 11.899417190512075, 11.825077691146884, 11.768135181966613, 11.704857584624463, 11.645346250044263, 11.607591513731755, 11.545679457058927, 11.505774541465644, 11.43888294167386, 11.415109242616566, 11.35902911211939, 11.307095578575236, 11.285896821096067, 11.246631802053958, 11.20644724473627, 11.166691646985615, 11.13819758875689, 11.088559754244974, 11.029769412948358, 11.024753032939374, 10.997180865407557, 10.956432553621287, 10.934295491344379, 10.905916012274313, 10.86421278032399, 10.862526170106012, 10.727449629583496, 10.731379770522059, 10.756320195457814, 10.765298854371746, 10.729341457897588, 10.699896427340136, 24.875535291389482, 24.91659364416988, 24.972935593782502, 22.57155993763013, 10.380811542724432, 10.395730970088774, 10.422300007375345, 10.442753308840711, 10.486979096691265, 25.110872814965134, 25.186577826460386, 14.181663435692489, 14.134264197869243, 14.09516005260409, 14.064456514707878, 14.022268190096465, 13.999346473254125, 10.051155071108493, 10.068941324290217, 10.089674309806629, 10.122777911439345, 13.807540535184366, 13.794727216534323, 13.765567198073512, 13.734183131510328, 13.70852218514272, 13.677469817554524, 13.644186721841592, 13.603837239391492, 13.577330036784797, 13.543773182775585, 13.520962728867364, 9.72499967086807, 9.740035304005, 9.758194717174412, 9.777864458736019, 9.802355628227705, 13.318267759421527, 13.293218899578473, 13.267657712282912, 13.256596715481987, 13.275221266952077, 13.295275828773566, 13.30668217625034, 13.273947238183187, 13.186558235719449, 13.10004379918366, 13.073948474099002, 13.055908760539523, 13.0425756781889, 9.397888177194826, 9.3931914575453, 9.40378097256777, 9.422866060888756, 9.4383880620241, 9.45379319709904, 13.072353754013193, 13.092895183385075, 13.1394717053182, 13.175450176289367, 13.228875738854885, 13.2611124676265, 13.314391598205951, 13.372929289604343, 13.426115671562577, 13.479246270011682, 13.555485093408116, 13.610334880624986, 13.68123859458349, 13.752154929821948, 13.817687929792854, 13.885005708519053, 13.959532208171854, 14.039500397125167, 9.071367987849387, 9.079423158222816, 9.087353682774815, 9.100630121237437, 9.117457474268083, 15.808646673646365, 15.786689972827848, 15.707356501850722, 15.671585230400797, 15.668559432044098, 15.644878313415813, 15.637454918554159, 15.694593767848815, 15.749763246695274, 15.73968288391967, 15.695704661461221, 15.655003364263969, 15.64939557911347, 15.662199553700354, 15.603441179287458, 15.581782553671822, 15.582346999095638, 15.586389194895453, 15.512735567801055, 15.495298588079987, 15.492672347378981, 15.514408679055848, 15.61379887033354, 15.694168520358442, 15.770670600529087, 8.740001487067886, 8.741703643517049, 8.74711188996545, 8.754326471144221, 8.759519570339492, 8.776124369417335, 18.293759933245898, 18.402847570430634, 16.661699864190766, 18.562935462971822, 18.451512511170325, 16.734202183392497, 16.73014406732511, 18.344402180468244, 18.31435606839477, 16.66372419649085, 18.124751806382978, 18.099258245632658, 18.014936718386622, 17.912578645858538, 17.840952730044286, 17.733703442453766, 17.653337893167866, 17.58623153449505, 17.54614535577762, 17.574348970988616, 17.565006229861453, 16.5100280478172, 16.42841952579392, 16.303113778698087, 16.063108479038217, 14.909850375704156, 14.81389811234564, 8.436329091579447, 8.424127111007575, 8.423666070264872, 8.427058235668177, 8.428373486499531, 8.435530204493784, 8.450520934617014, 14.842401076113898, 14.89455385185651, 14.986238389424926, 15.006290970584672, 15.294283776990511, 15.341671109119055, 15.406776930077093, 15.517492938758753, 16.40080962717225, 16.334211429832397, 16.319131724630754, 16.25593766919573, 16.208406395927742, 16.20049829796005, 14.310375359014753, 14.187654381185723, 14.116575358818316, 14.151108524643199, 14.225403651372392, 15.92597142435152, 15.864305901690848, 8.035113738416477, 8.039788287747692, 8.010385315284825, 8.006879623492212, 8.009282644186602, 8.01359614018387, 13.600000000000001, 13.541902503541763, 13.549609711407754, 13.60111740266742, 13.67641938033303, 8.12285201863348, 8.10835173313243, 8.099760303197897, 8.093078406383583, 8.104293206245394, 8.109418138695062, 8.108456132538553, 13.428100741480886, 13.453643289568237, 13.492952561484106, 13.454212402876028, 13.439241006840852, 7.851449844794053, 7.845943041823064, 7.83636616736981, 7.832685876317442, 7.828920810609562, 7.823080325380461, 7.817157072859139, 7.815129404971961, 7.8110276628528865, 7.7988933625035886, 7.792641699264086, 7.776383143902362, 7.769974303256796, 7.759518986459399, 7.7470061474723275, 7.734420411824751, 7.735617515725762, 7.728813036134663, 7.729836289916503, 13.368494944026835, 13.357492975248764, 13.419290271771995, 14.618125782222965, 14.605593004580147, 14.610563778746467, 14.583833319203944, 13.440853005322712, 13.54033477772603, 13.570783456382628, 13.532373765650703, 13.564312733528375, 13.836505789880604, 13.791276892510805, 14.338924383515344, 14.193711468888111, 13.366590936829834, 13.217684624423146, 13.145917068920813, 13.099101728395222, 13.125150209785595, 13.246795929522634, 13.256827009648461, 13.241744242991718, 13.207376903798856, 13.211026552175575, 13.225869023882247, 12.53285666019335, 12.679228570369737, 12.678920949989312, 12.636731076821743, 12.637941452618854, 12.640816767766207, 12.641577176723487, 12.63270136728217, 12.627388953920924, 12.578712312273368, 12.552447885395672, 12.524173708342818, 12.49763436185043, 12.485869559651263, 12.49996891220626, 12.487784097009072, 12.492100734175128, 12.462850989773909, 12.405756672431242, 12.394745982613994, 12.368813816213443, 12.38316990353201, 12.334875852842242, 12.29201997086945, 12.30938530327133, 12.368385285417723, 12.496068603478346, 7.523394287590789, 7.509334246944629, 7.487995719383353, 7.470232848063581, 7.461416434365143, 7.450727047813282, 7.448915700386988, 7.450566128974964, 7.468128520153185, 7.45348808502136, 12.257035393433682, 12.222445360902388, 12.182452784160805, 12.147666574534892, 12.125081445351455, 12.104090080814792, 12.088178817336647, 12.056369926982594, 12.045334032804114, 12.053180447679534, 12.04685657822283, 12.057564351762164, 11.988668453892348, 11.653952512642785, 12.021810904605399, 11.495577259771533, 11.53651165130702, 11.52945872510196, 11.500176959241724, 11.452221715227353, 11.43789348944346, 11.43342716793472, 11.411975711723269, 11.375350300898457, 11.343637029414822, 7.203108891589137, 7.198197256883821, 7.193172115050403, 7.178173547087012, 7.169674257221198, 7.170880971466358, 7.158907557008952, 7.151730118405949, 7.137976621314751, 7.1402892055217535, 7.140828080029065, 7.139608270415563, 7.139839532307382, 7.1271776281864625, 7.1223763935231705, 7.112705124592812, 7.099787853891613, 7.089939508430475, 7.090953911793093, 7.0684018223048035, 7.056723577682998, 7.0449628267814495, 7.037749481930115, 7.028882885556279, 7.019911815785757, 7.010836268082656, 7.00621867633455, 6.993886863856627, 6.987511008968465, 6.978000338187158, 6.9638913860997995, 6.95269690830208, 6.758589373208333, 6.736347570046814, 6.725960855259958, 6.718067541040543, 6.710016946865261, 6.696613292766861, 6.688274149247702, 6.681062826951197, 6.6762379304574875, 6.664853785269372, 6.660930705324086, 6.642949917256736, 6.63992764757414, 6.624228159644888, 6.619581756199331, 6.613490060202693, 6.60352444306589, 6.592181808079162, 6.579482827216402, 6.57267009590084, 6.5656556699146575, 6.5536806435298365, 6.543924730922612, 6.536345599122357, 6.526226653649912, 6.513610156904341, 6.499692933566424, 6.486790680366411, 6.4560847471888945, 6.442305237958869, 6.426171084807498, 6.424174821804469, 6.4098888899358055, 6.323787311059686, 6.299551725097761, 6.298462711374972, 6.2909999999999995, 6.271344424007145, 6.259465596221837, 6.247363328709631, 6.236007060211818, 6.224411715029876, 6.214485707665689, 6.20334283851183, 6.191005883635515, 6.18215388081244, 6.16561189373662, 6.155301734669344, 6.144704471368, 6.130218997243393, 6.114615805096674, 6.1014565638471545, 6.089793978165689, 6.075236304299416, 6.059576130541174, 6.045396410005784, 6.044482991744102, 6.022962932943431, 6.011264420486492, 5.8583285485679095, 5.846450523280419, 5.826918002913969, 5.810009118615286, 5.792083161275935, 5.77946825931703, 5.765737914620062, 5.746128065065183, 5.728945369007917, 5.7134235922601615, 5.696191609769938, 5.683158890626386, 5.665151585700664, 5.649958285336112, 5.626807082174258, 5.605884812025858, 5.5242987974589015, 5.43256224110449, 5.408984277524045, 5.382975674985088, 5.362784984361184, 5.342600073076135, 5.321410842354092, 5.299726389026853, 5.276595880584454, 5.255805258384775, 5.23124249391226, 5.21073425559679, 5.18343191047349, 5.16181355909556, 5.067197370674036, 4.995876535391415, 4.967455058253151, 4.938504166723135, 4.910413199683115, 4.882401763965287, 4.85408825678414, 4.82705437323635, 4.7967649615049295, 4.764948209008901, 4.735820619713039, 4.710532474173292, 4.680318815321927, 4.6188366461914, 4.584453107864473, 4.551841895457675, 4.516276988893702, 4.480935926026804, 4.445714990942075, 4.411137564535158, 4.374216396604682, 4.333408903673053, 4.302857740550891, 4.262025088448651, 4.146615391992245, 4.100943831530048, 4.057499042743517, 4.013291135925271, 3.9689748932478555, 3.92216984781612, 3.876601148569508, 3.8298883177141017, 3.781403860837697, 3.7354759198538083, 3.6833804948361126, 3.6333372597524534, 3.581062978785286, 3.526078472988569, 3.471892569042897, 3.4155742361404635, 3.3000000000000007, 3.239594346261967, 3.178421907436656, 3.1163267949428946, 3.055526690626536, 2.8830271406330836, 2.7727384038186154, 2.7010522507796533, 2.629657254969518, 2.6228366940497567, 2.317606901805088, 2.242431400348589, 2.161574348495882, 2.079877817422951]
  out "xl":dbl[](array[numeric])
  out "yl":dbl[](array[numeric])
  out "xr":dbl[](array[numeric])
  out "yr":dbl[](array[numeric])
  out "size(s) 3":i32=273
  out "size(s) 4":i32=233
  out "size limit":i32=74
  out "h_lf":dbl[](array[numeric])=[-1.07768170874119, -0.9500104358126387, -0.8152801995859489, -0.6832149509832309, -0.5579658214676491, -0.43634713174659895, -0.3636177945739105, -0.4219341557757026, -0.43418280012028193, -0.4285800458197435, -0.47492259541262927, -0.43011998989542144, -0.448140819410384, -0.42370272779821094, -0.4351070943600193, -0.3916639450286278, -0.3566256576667743, -0.31695052117940714, -0.29608961933059963, -0.29070058934802034, -0.19489158382745403, -0.13694705181123534, -0.0036604327923040465, 0.15093015758716827, 0.15093015758716827, 0.24134113354650677, 0.4371774287913892, 0.4371774287913892, 0.5886484511821607, 0.7188655986278671, 0.8431460626855709, 0.9539279580870911, 1.0615621391385646, 1.1504547666405178, 1.1293783256575063, 1.1293783256589616, 1.129378308345949, 1.1293783256589178, 1.2328992187190753, 1.2383213544784377, 1.2299347078478895, 1.2485889663962422, 1.2485889663962422, 1.2492445630317817, 1.2507974714580428, 1.2535353037498, 1.2548915682041502, 1.2388573722116965, 1.2551948137598792, 1.2561989169947274, 1.2545138672661875, 1.2372556012572844, 1.2374470995854208, 1.2497004386998842, 1.258883376955003, 1.238295612670253, 1.249261743063205, 1.2490590423907508, 1.2394351036162379, 1.249147146451496, 1.2523281510667994, 1.2568185177320512, 1.2637485927398984, 1.2729524270473782, 1.2872258426538232, 1.3082533285080937, 1.3356267808199382, 1.3717983894543175, 1.4090203881905266, 1.4509264137298254, 1.496939359193244, 1.5483512846148995, 1.5906635102611244, 1.5906635102611244, 1.5906635102611244, 1.5906635102611244, 1.5906635102611244, 1.5906635102611244, 1.5906635102611244, 1.5906635102611244, 1.5906635102611244]
  out "h_rf":dbl[](array[numeric])=[-0.8152801995859489, -0.6832149509832309, -0.5579658214676491, -0.43634713174659895, -0.3636177945739105, -0.38220962901672345, -0.4254071654192556, -0.43418280012028193, -0.4285800458197435, -0.47492259541262927, -0.47492259541262927, -0.43011998989542144, -0.448140819410384, -0.42370272779821094, -0.4351070943600193, -0.3916639450286278, -0.3566256576667743, -0.29608961933059963, -0.29070058934802034, -0.19489158382745403, -0.13694705181123534, -0.0036604327923040465, 0.15093015758716827, 0.24134113354650677, 0.4371774287913892, 0.5886484511821607, 0.5886484511821607, 0.7188655986278671, 0.8431460626855709, 0.9539279580870911, 1.0615621391385646, 1.142586619661877, 1.1504547666405178, 1.1293783256600938, 1.1293783256589616, 1.129378308345949, 1.1293783256583803, 1.1293783256589178, 1.2328992187190753, 1.2383213544784377, 1.2299347078478895, 1.2485889663962422, 1.2492445630317817, 1.2507974714580428, 1.2535353037498, 1.2548915682041502, 1.2548915682041502, 1.2388573722116965, 1.2551948137598792, 1.2561989169947274, 1.2545138672661875, 1.2372556012572844, 1.2374470995854208, 1.2497004386998842, 1.258883376955003, 1.238295612670253, 1.249261743063205, 1.2490590423907508, 1.2394351036162379, 1.249147146451496, 1.2523281510667994, 1.2568185177320512, 1.2637485927398984, 1.2729524270473782, 1.2872258426538232, 1.3082533285080937, 1.3356267808199382, 1.3717983894543175, 1.4509264137298254, 1.496939359193244, 1.5483512846148995, 1.5906635102611244, 1.5906635102611244, 1.5906635102611244, 1.5906635102611244, 1.5906635102611244, 1.5906635102611244, 1.5906635102611244, 1.5906635102611244, 1.5906635102611244, 1.5906635102611244]
  out "idxfront":i32=29
  out "x_lf":dbl[](array[numeric])=[4.268405081027962, 3.621683915224116, 3.047106041353469, 2.510462912500592, 2.0491128435969053, 1.6717803031765444, 1.382142960309996, 1.1959993160946079, 1.1054006303411974, 1.0979165970842675, 1.1737168928660435, 1.1843207893936691, 0.9474282855978409, 0.6385020552290817, 0.419575244320852, 0.1838352755824535, -0.009964744332359832, -0.35518195016074827, -0.45298194084737164, -0.7176786200112701, -0.8688385259169258, -1.1085156622100212, -1.1880415455459132, -1.2704725759207889, -1.3184121361781558, -1.4069677759384254, -1.5360201682793213, -1.3561071997832572, -1.2510471183409675, -0.8366356389407819, -0.25840338682322134, 0.16096387556169744, 1.0225238690494292, 1.789749584208254, 2.5228442391661003, 3.2582102778678763, 3.9651965467946226, 4.668134133038354, 5.307553335275859, 5.78252262984093, 6.192213941390776, 6.6118249613773, 7.031435981354307, 7.451046959879165, 7.870658023263255, 8.29026904324418, 8.941462638036167, 9.425515144535234, 9.885483743848654, 10.401757606348562, 10.881711564834836, 11.36208862651888, 11.863127252302835, 12.361307835200675, 12.818353134972247, 13.324432307326454, 13.824206750930301, 14.31718322119306, 14.784287511760091, 15.263954206446822, 15.767174370388378, 16.292185876084783, 16.75852144103834, 17.267766359662545, 17.768273946512444, 18.22690912729219, 18.730869971236952, 19.225262001281948, 19.734216994347804, 20.230432724257977, 20.735913809073367, 21.2561960050937, 21.788791728779202, 22.326632476864347, 22.876721241835906, 23.429244142571054, 23.98770499081292, 24.554787387138468, 25.118391588340955, 25.673660066590077, 26.18065040856573]
  out "y_lf":dbl[](array[numeric])=[-12.88508999526141, -12.476353054215982, -12.103977464857248, -11.548148209415558, -10.930894805835154, -10.26756057127472, -9.568776800965319, -8.814645985482116, -8.049202785958764, -7.296671194766963, -6.557761176836454, -5.938710822442266, -5.509159445818854, -5.132715472009396, -4.676378026833698, -4.234658759524203, -3.7673976963609204, -3.421964929853629, -2.867382717507443, -2.449953337988509, -1.9262536967618593, -1.4973315043056692, -0.9430014105996793, -0.40241467019349075, 0.14866852309460077, 0.6669091172252917, 1.1583339490694162, 1.8062723733121595, 2.388292629561391, 3.041332836906522, 3.6462076206641867, 4.157380552096733, 4.573336958069159, 4.872028835248066, 5.091117493868304, 5.224453014781301, 5.298985470194547, 5.303829930891121, 5.314489619988054, 5.499260342882392, 5.767578377538095, 5.965850444112123, 6.164122510695547, 6.362394628537478, 6.560666653667127, 6.758938720246449, 6.638430091943965, 6.7872346473437695, 6.978852871826557, 7.088582585204193, 7.246253367993072, 7.400215653030386, 7.555578647491765, 7.71387478720567, 7.925551006627789, 8.035929820683164, 8.195204964883214, 8.362176683901211, 8.582089160559374, 8.747536982716873, 8.873738921644886, 9.01251449475196, 9.242709401695103, 9.375580399508735, 9.543086650041982, 9.733448334959586, 9.868788167121654, 10.021119094451475, 10.171413059138207, 10.30556202953376, 10.430073101962705, 10.534448967040744, 10.608420742432445, 10.647751914269572, 10.641356408970907, 10.611684524318402, 10.544968307804066, 10.440894542675338, 10.29074396046648, 10.145855393258826, 10.13578159769189]
  out "y_lr":dbl[](array[numeric])=[-12.394475085925853, -12.468848004172973, -12.46556121048128, -12.396862894746317, -12.246368091793784, -12.019035975405181, -11.720972823852813, -11.351604480539473, -10.9187272965521, -10.435506568927917, -9.911076816611818, -9.396790932425702, -8.94217770417287, -8.508220146433779, -8.046599893138712, -7.591350988647731, -7.132757747412678, -6.712478970349138, -6.230370892043438, -5.78459397102167, -5.299073273182397, -4.852583658065757, -4.362819528952363, -3.8696113626030337, -3.3670354649567713, -2.872084563711297, -2.3864262804699528, -1.8236817101647458, -1.2770657460100523, -0.6586423753999348, -0.011729481392127039, 0.5646128034759201, 1.2213208404472837, 1.7947689198701726, 2.3066704610229336, 2.7635207341691057, 3.1585963413975073, 3.5000475733509786, 3.7780911847511787, 3.989392817832373, 4.186857068929599, 4.385129135512282, 4.583401202091919, 4.781673262015884, 4.979945345061554, 5.178217411642675, 5.411865865207488, 5.579615837371853, 5.741945596749875, 5.916936525444208, 6.076908437454078, 6.236323399004274, 6.401306482512538, 6.564371420870169, 6.719807026979052, 6.887492993910782, 7.050300405025509, 7.21134506013289, 7.370743694649158, 7.536861034317964, 7.705994400600314, 7.877059073726956, 8.035000563275199, 8.2062957772499, 8.37309049525761, 8.529725475528517, 8.699101274794145, 8.862604212457192, 9.028688726984386, 9.187252683732133, 9.344272137557052, 9.499243309177244, 9.648132932035574, 9.785622802458096, 9.90991397952625, 10.015721049186642, 10.102511004881439, 10.167872136725581, 10.20770427709779, 10.219359136478959, 10.209285340912023]
  out "x_lr":dbl[](array[numeric])=[7.935733401581995, 7.3216763036249155, 6.729395708788731, 6.11180757566516, 5.507368188988451, 4.930972520387127, 4.391802788109021, 3.8892949913512833, 3.4411722551162045, 3.0569246353311437, 2.7374541534178105, 2.500254660428585, 2.3274230818952644, 2.1537473135747893, 1.946534501105246, 1.740311192177928, 1.5276801193422518, 1.3367156085885759, 1.0898435638455792, 0.885496931363002, 0.6523741827186508, 0.45106216037155633, 0.22434793239093076, 0.02124995471198088, -0.16523154823900843, -0.32737353443336026, -0.47551325407460976, -0.6395645619386285, -0.7459253719982921, -0.8230920678538325, -0.8147271750975142, -0.7233550174119514, -0.5439971002335124, -0.26462901118463134, 0.08627806496138235, 0.49527482617146334, 0.9471285592689194, 1.4375971487852823, 1.9416240656384702, 2.404609064220973, 2.8468708880536386, 3.2664819080360727, 3.6860929280148693, 4.105703933906775, 4.525314969924736, 4.94492598990481, 5.45068332709565, 5.928136581982702, 6.39835592960634, 6.892164252318939, 7.371350837869192, 7.849916247346979, 8.347781498446727, 8.844399816673128, 9.320327769778217, 9.807175868720792, 10.30579893647544, 10.800709622012374, 11.288197958814006, 11.767632746974252, 12.256280932305932, 12.770717292259999, 13.261173965936324, 13.7573855438323, 14.258130217576293, 14.72818774974823, 15.22062317451208, 15.711312191139838, 16.21510047159616, 16.703481603659235, 17.198819483826192, 17.703964418340465, 18.21557926361523, 18.72847553273765, 19.249740131820566, 19.777555829433023, 20.314255449157223, 20.86487427625775, 21.41932354206416, 21.974390246783386, 22.481380588759038]
  out "x_rf":dbl[](array[numeric])=[4.029727557567421, 3.6180328097977874, 3.223011647332728, 2.9233511377966357, 2.689072820549753, 2.5238494186994718, 2.429157241714723, 2.4301953407171064, 2.5013855273866046, 2.6249175899193253, 2.8050596365405447, 2.866630032088314, 2.6175452761484426, 2.2806394644085106, 2.0591426387395075, 1.816820684345251, 1.6272374426657925, 1.2456086641343638, 1.1830663602782474, 0.9045789852481053, 0.7719926193687411, 0.5237691693489401, 0.4756537552743114, 0.4162717609270965, 0.3919303444954846, 0.31470482559829327, 0.18845778122631784, 0.40981640839469646, 0.5321001995045994, 0.9633523021812784, 1.521133581744715, 1.9087968343502006, 2.653234412757369, 3.286794948446148, 3.8774400929827664, 4.455420576544079, 5.0064669337769665, 5.5456498745443685, 6.054990411877582, 6.5170527771625615, 6.9612134969300445, 7.380824516912359, 7.800435536891207, 8.220046543592373, 8.639657578801101, 9.05926859878115, 9.53816955915121, 10.013005376413464, 10.487222418210283, 10.971747581366934, 11.450582071583536, 11.92830647982888, 12.424665062292728, 12.92052568909362, 13.404931287233795, 13.88313130413464, 14.381187347617834, 14.877047254377649, 15.373590711392088, 15.852931694857102, 16.335266299545196, 16.844569594421273, 17.346055470539916, 17.836607527247924, 18.33746126505619, 18.812504031880277, 19.299906837774657, 19.788863835765653, 20.290136939719932, 20.774475108702013, 21.26414130527071, 21.759809568378643, 22.255958771674976, 22.746046639367226, 23.232558099403576, 23.71917231966218, 24.202954489532033, 24.687609098141053, 25.158789272141938, 25.637901488807312, 26.144891830782964]
  out "y_rf":dbl[](array[numeric])=[-11.100984325802692, -10.676356757156134, -10.312593302321174, -9.796142697605768, -9.24850031348251, -8.68200760073984, -8.104617965819848, -7.504394035357247, -6.912881454987139, -6.343640257241457, -5.7970241311626225, -5.298526777073928, -4.837810625998486, -4.395569130111484, -3.9335329829926415, -3.477454259558837, -3.019354249167866, -2.5988796310026063, -2.116818958467629, -1.6700300967794037, -1.1862042709391463, -0.7386179689957126, -0.2558930159277013, 0.22599088524947808, 0.7096752956055377, 1.1921171266061346, 1.6742562316554923, 2.1548606836149524, 2.6340275331875573, 3.0479216012190924, 3.3755636155577737, 3.727171360920363, 3.8112456757152957, 3.8726014104623374, 3.9057609766876302, 3.8803222544965603, 3.830736178965827, 3.732217343957194, 3.6770105158401343, 3.8559510406889004, 4.140114189428136, 4.338386256000174, 4.5366583225844686, 4.734930453740099, 4.933202465556496, 5.131474532135405, 4.940213129864795, 5.08580723853443, 5.282412313546512, 5.381212845405997, 5.538510311631407, 5.691591252352165, 5.845410442913117, 6.002946561976053, 6.223808937073938, 6.324832093793923, 6.483547109202469, 6.65145979781331, 6.881288837504521, 7.046623840270758, 7.1657367085236965, 7.2993676161344965, 7.541297116510339, 7.667827570185912, 7.835449160289259, 8.031367664803067, 8.161100536282527, 8.311629997625584, 8.459410426448219, 8.589747970864101, 8.709324511301917, 8.806336303214847, 8.870101164785106, 8.897297184694423, 8.876879112206687, 8.835187507116117, 8.757884746998592, 8.645801677922556, 8.49119734335885, 8.34621061605557, 8.336136820488635]
  out "y_rr":dbl[](array[numeric])=[-10.610369416467135, -10.668851707113124, -10.674177047945207, -10.644857382936525, -10.563973599441141, -10.433483004870304, -10.256813988707341, -10.041352530414605, -9.782405965580475, -9.482475631402409, -9.150339770937986, -8.756606887057366, -8.2708288843525, -7.771073804535867, -7.303754849297656, -6.834146488682364, -6.384714300219623, -5.889393671498115, -5.479807133003624, -5.004670729812564, -4.559023847359684, -4.0938701227558, -3.675711134280385, -3.241205807160065, -2.8060286924458344, -2.346876554330454, -1.8705039978838767, -1.4750933998619535, -1.0313308423838858, -0.6520536110873648, -0.2823734864985398, 0.13440361229955045, 0.45922955809342025, 0.7953414950844444, 1.1213139438422601, 1.4193899738843643, 1.690347050168787, 1.9284349864170522, 2.14061208060326, 2.34608351563888, 2.55939288081964, 2.7576649474003334, 2.955937013980841, 3.154209087218505, 3.3524811569509234, 3.55075322353163, 3.713648903128317, 3.8781884285625137, 4.0455050384698295, 4.209566785646012, 4.369165381092413, 4.527698998326052, 4.6911382779338915, 4.853443195640552, 5.0180649574252, 5.176395267021541, 5.338642549344766, 5.500628174044989, 5.669943371594305, 5.835947891871848, 5.997992187479124, 6.163912195109493, 6.333588278090435, 6.4985429479270795, 6.6654530055048875, 6.827644805371998, 6.99141364395502, 7.1531151156313015, 7.316686094294399, 7.471438625062473, 7.623523546896266, 7.771130645351347, 7.909813354388237, 8.035168072882946, 8.14543668276203, 8.239224031984357, 8.315427444075965, 8.3727792719728, 8.40815765999016, 8.419714359275703, 8.409640563708768]
  out "x_rr":dbl[](array[numeric])=[7.6970558781214535, 7.318025198198587, 6.905301314767991, 6.5246958009612035, 6.1473281659413, 5.783041635910055, 5.438817069513747, 5.123491015973782, 4.837157152161612, 4.5839256281662015, 4.368796897092311, 4.1825639031232305, 3.997540072445866, 3.7958847227542183, 3.5861018955239015, 3.3732966009407255, 3.164882306340404, 2.9375062228836883, 2.725891864971198, 2.5077545366223775, 2.2932053280043174, 2.083346991930518, 1.8880432332111552, 1.7079942915598665, 1.545110932434632, 1.3942990671033586, 1.2489646954310292, 1.1263590462393254, 1.0372219458472747, 0.9768958732682278, 0.9648097934704221, 1.024477941376552, 1.0867134434744272, 1.2324163530532624, 1.4408739187780488, 1.6924851248476664, 1.9883989462512632, 2.3151128902912976, 2.689061142240193, 3.139139211542605, 3.6158704435929074, 4.035481463571131, 4.45509248355177, 4.8747035176199836, 5.294314525462582, 5.713925545441782, 6.047390248210693, 6.515626813860932, 7.000094603967969, 7.462154227337311, 7.940221344617893, 8.41613410065698, 8.90931930843662, 9.403617670566074, 9.906905922039765, 10.365874865528978, 10.862779533162971, 11.360573655196962, 11.877501158446002, 12.356610235384531, 12.82437286146275, 13.323101010596488, 13.8487079954379, 14.326226711417679, 14.82731753612004, 15.313782654336318, 15.789660041049787, 16.27491402562354, 16.77102041696829, 17.247523988103268, 17.727046980023538, 18.20757798162541, 18.682746306511003, 19.147889695240533, 19.60557698938824, 20.06748400652415, 20.52950494787634, 20.997695987260336, 21.45972122586514, 21.93863166900062, 22.445622010976273]
  out "y_path":dbl[](array[numeric])=[-11.502422251196494, -11.568849855643048, -11.569869129213243, -11.520860138841421, -11.405170845617462, -11.226259490137743, -10.988893406280077, -10.696478505477039, -10.350566631066288, -9.958991100165163, -9.530708293774902, -9.076698909741534, -8.606503294262685, -8.139646975484823, -7.675177371218184, -7.212748738665048, -6.758736023816151, -6.300936320923626, -5.855089012523531, -5.394632350417117, -4.92904856027104, -4.473226890410778, -4.019265331616374, -3.5554085848815493, -3.086532078701303, -2.6094805590208754, -2.1284651391769147, -1.6493875550133497, -1.154198294196969, -0.6553479932436498, -0.14705148394533343, 0.3495082078877353, 0.840275199270352, 1.2950552074773085, 1.7139922024325969, 2.091455354026735, 2.424471695783147, 2.7142412798840154, 2.9593516326772193, 3.1677381667356266, 3.373124974874619, 3.571397041456308, 3.76966910803638, 3.9679411746171946, 4.166213251006239, 4.364485317587152, 4.562757384167902, 4.728902132967184, 4.893725317609852, 5.06325165554511, 5.223036909273246, 5.382011198665163, 5.546222380223215, 5.708907308255361, 5.868935992202126, 6.031944130466162, 6.194471477185138, 6.35598661708894, 6.520343533121731, 6.686404463094906, 6.851993294039719, 7.0204856344182245, 7.184294420682817, 7.35241936258849, 7.5192717503812485, 7.678685140450257, 7.845257459374583, 8.007859664044247, 8.172687410639393, 8.329345654397303, 8.483897842226659, 8.635186977264295, 8.778973143211905, 8.910395437670521, 9.02767533114414, 9.127472540585499, 9.208969224478702, 9.27032570434919, 9.307930968543975, 9.319536747877331, 9.309462952310396]
  out "x_path":dbl[](array[numeric])=[7.816394639851724, 7.319850750911751, 6.817348511778361, 6.318251688313182, 5.827348177464875, 5.357007078148591, 4.915309928811384, 4.506393003662533, 4.139164703638908, 3.8204251317486726, 3.553125525255061, 3.3414092817759076, 3.162481577170565, 2.974816018164504, 2.7663181983145737, 2.5568038965593267, 2.346281212841328, 2.137110915736132, 1.9078677144083886, 1.6966257339926898, 1.4727897553614842, 1.267204576151037, 1.056195582801043, 0.8646221231359237, 0.6899396920978118, 0.5334627663349991, 0.38672572067820976, 0.24339724215034841, 0.1456482869244913, 0.07690190270719764, 0.07504130918645387, 0.15056146198230025, 0.2713581716204574, 0.48389367093431557, 0.7635759918697156, 1.093879975509565, 1.4677637527600913, 1.8763550195382899, 2.3153426039393317, 2.771874137881789, 3.231370665823273, 3.6509816858036017, 4.070592705783319, 4.490203725763379, 4.909814747693659, 5.329425767673296, 5.749036787653171, 6.221881697921817, 6.699225266787154, 7.177159239828125, 7.6557860912435425, 8.133025174001979, 8.628550403441674, 9.124008743619601, 9.613616845908991, 10.086525367124885, 10.584289234819206, 11.080641638604668, 11.582849558630004, 12.062121491179392, 12.540326896884341, 13.046909151428244, 13.554940980687112, 14.041806127624989, 14.542723876848166, 15.020985202042274, 15.505141607780933, 15.99311310838169, 16.493060444282225, 16.97550279588125, 17.462933231924865, 17.955771199982937, 18.449162785063116, 18.938182613989092, 19.427658560604403, 19.922519917978587, 20.42188019851678, 20.931285131759044, 21.43952238396465, 21.956510957892004, 22.463501299867655]
  out "h_path":dbl[](array[numeric])=[-1.7037866247771944, -1.5728247200893424, -1.4729147677282362, -1.3393532640375114, -1.2073117198254844, -1.07768170874119, -0.9500104358126387, -0.8152801995859489, -0.6832149509832309, -0.5579658214676491, -0.43634713174659895, -0.3636177945739105, -0.38220962901672345, -0.4219341557757026, -0.4254071654192556, -0.43418280012028193, -0.4285800458197435, -0.47492259541262927, -0.43011998989542144, -0.448140819410384, -0.42370272779821094, -0.4351070943600193, -0.3916639450286278, -0.3566256576667743, -0.31695052117940714, -0.29608961933059963, -0.29070058934802034, -0.19489158382745403, -0.13694705181123534, -0.0036604327923040465, 0.15093015758716827, 0.24134113354650677, 0.4371774287913892, 0.5886484511821607, 0.7188655986278671, 0.8431460626855709, 0.9539279580870911, 1.0615621391385646, 1.142586619661877, 1.1504547666405178, 1.1293783256575063, 1.1293783256600938, 1.1293783256589616, 1.129378308345949, 1.1293783256583803, 1.1293783256589178, 1.2328992187190753, 1.2383213544784377, 1.2299347078478895, 1.2485889663962422, 1.2492445630317817, 1.2507974714580428, 1.2535353037498, 1.2548915682041502, 1.2388573722116965, 1.2551948137598792, 1.2561989169947274, 1.2545138672661875, 1.2372556012572844, 1.2374470995854208, 1.2497004386998842, 1.258883376955003, 1.238295612670253, 1.249261743063205, 1.2490590423907508, 1.2394351036162379, 1.249147146451496, 1.2523281510667994, 1.2568185177320512, 1.2637485927398984, 1.2729524270473782, 1.2872258426538232, 1.3082533285080937, 1.3356267808199382, 1.3717983894543175, 1.4090203881905266, 1.4509264137298254, 1.496939359193244, 1.5483512846148995, 1.5906635102611244, 1.5906635102611244]
  out "R0":dbl=3.023957560629749
  out "element":dbl=2.140625
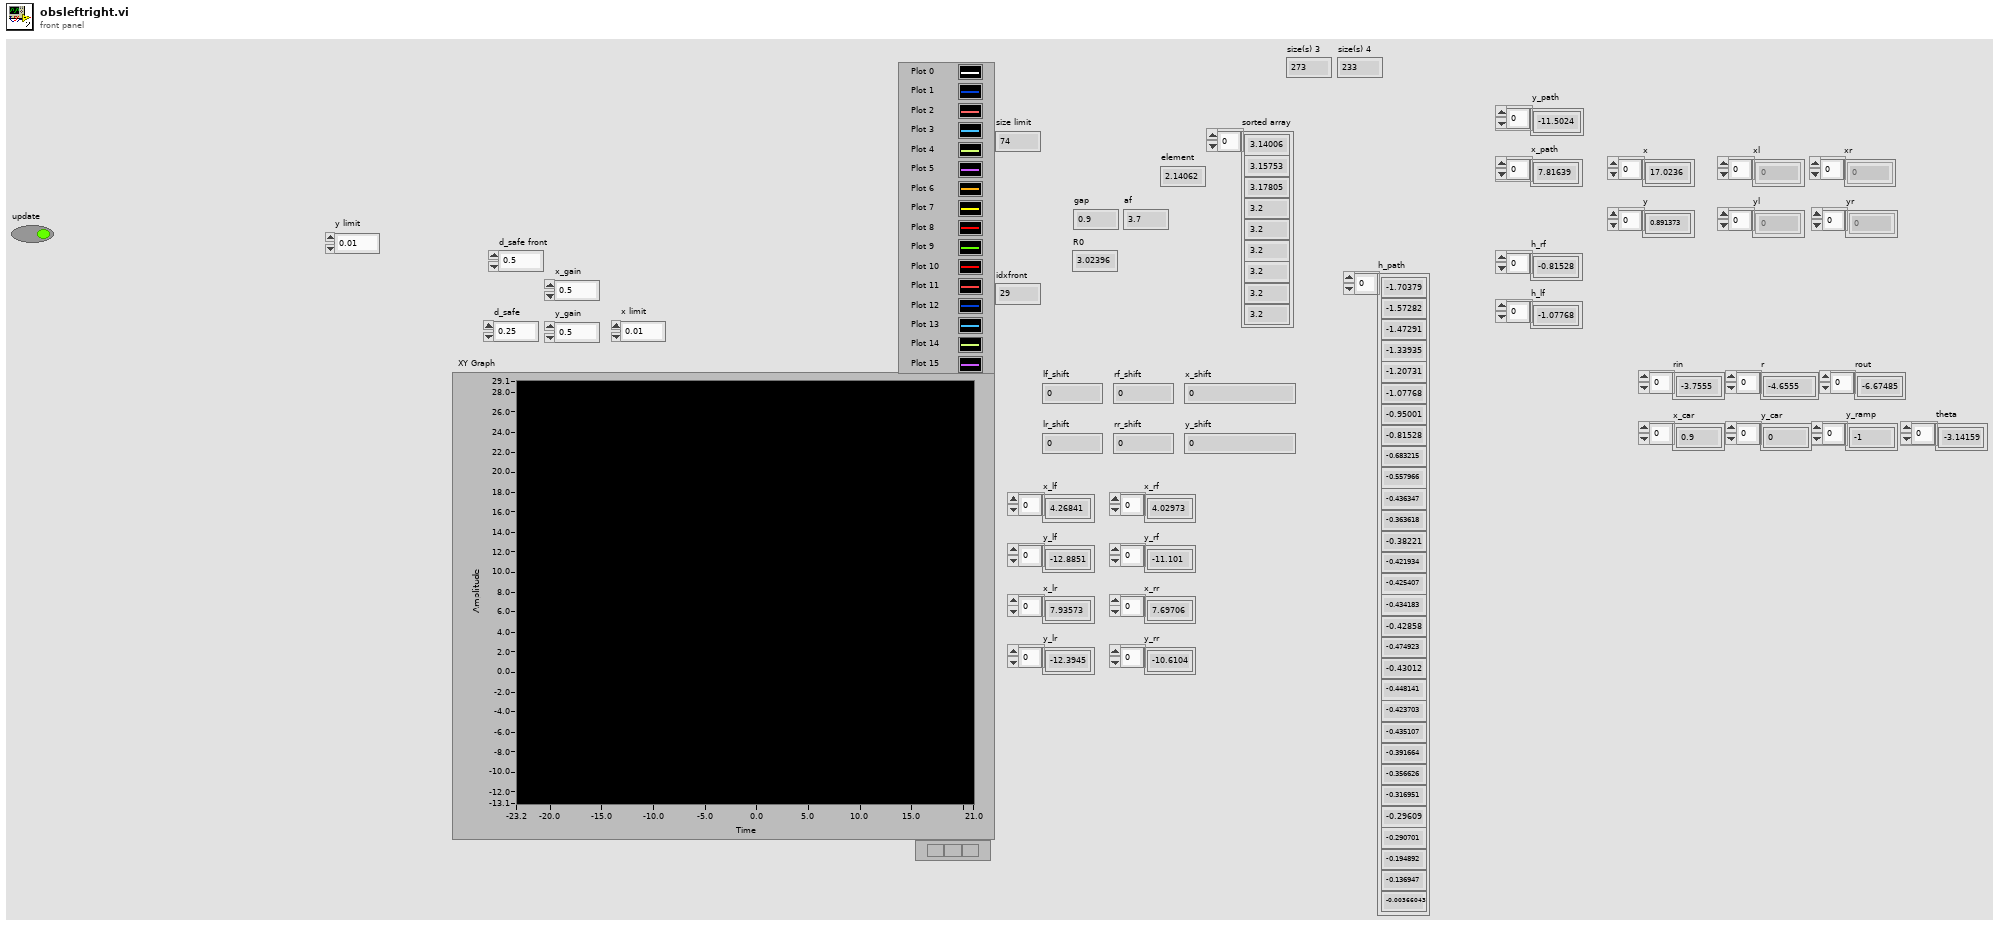
[diagram p1: front panel]
types:
  T1 = cluster{"C_Wheel base":dbl, "ratio_steer":dbl, "Overall width":dbl, "af":dbl, "turn radius":dbl, "eval":dbl, "ap":dbl, "an":dbl, "Vmax":dbl, "mu":dbl, "Vlast":dbl}
  T2 = cluster{"hash":i64, "sys time":i64, "size":i64, "x":dbl[], "y":dbl[], "point_flag":i32[]}
  T3 = cluster{"delta":bool, "element":dbl, "element":dbl}[]
  T4 = cluster{"element":bool, i32, "element":dbl, "element":dbl}[]
  T5 = cluster{bool, "Rotational position":dbl, "Rotational position":dbl}[]
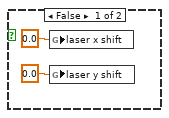
[diagram p2: hidden frame]
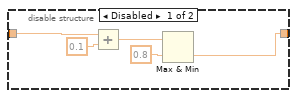
[diagram p4: hidden frame]
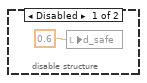
[diagram p5: hidden frame]
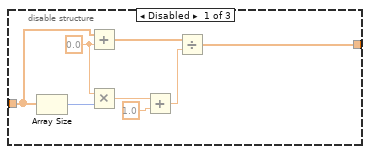
[diagram p6: hidden frame]
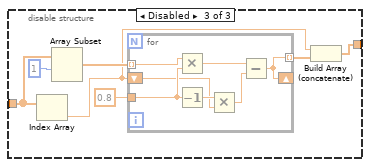
[diagram p7: hidden frame]
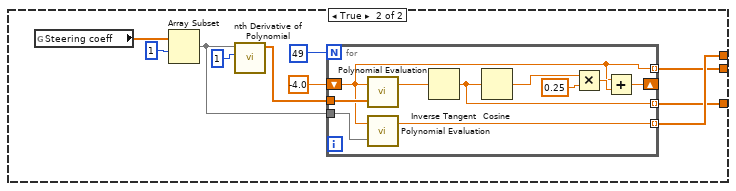
[diagram p9: hidden frame]
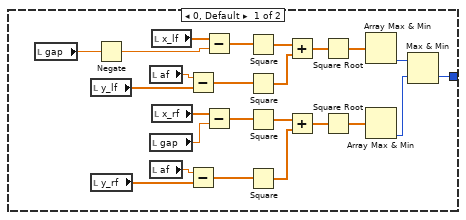
[diagram p10: hidden frame]
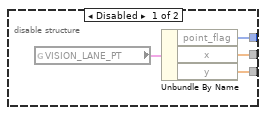
[diagram p11: hidden frame]
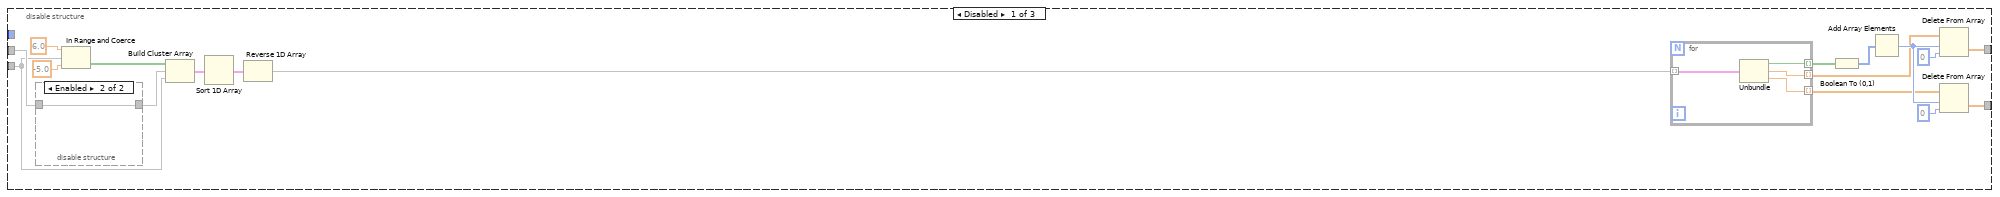
[diagram p12: hidden frame]
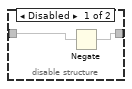
[diagram p13: hidden frame]
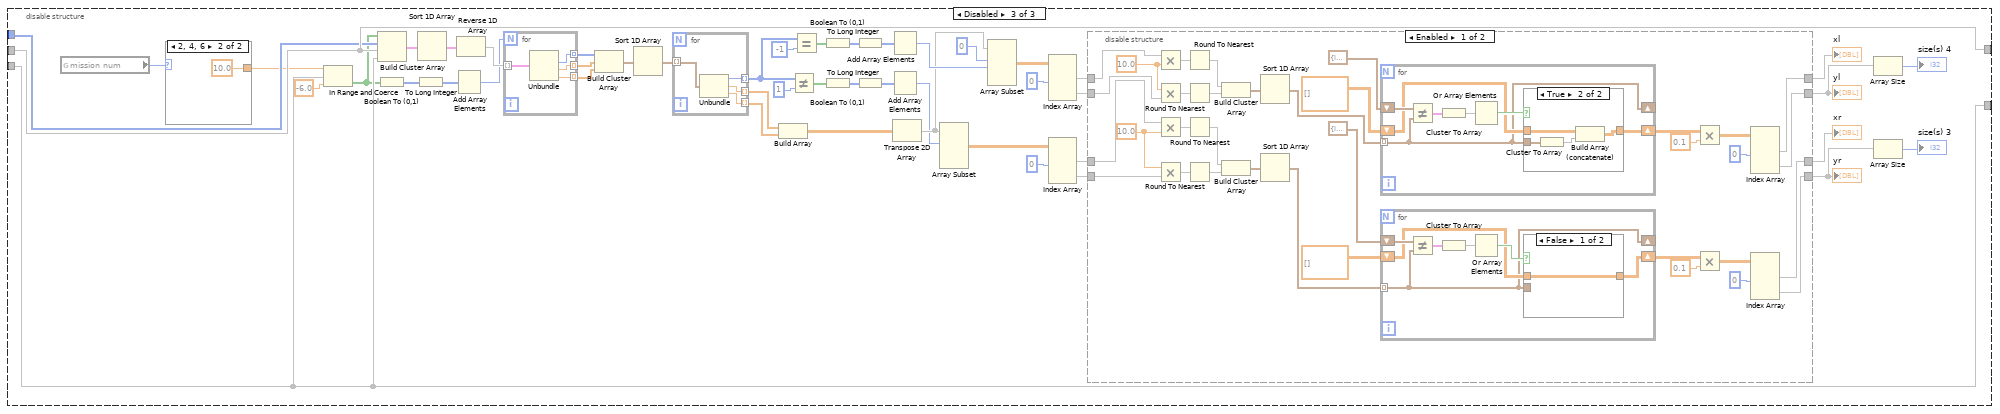
[diagram p14: hidden frame]
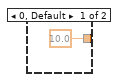
[diagram p15: hidden frame]
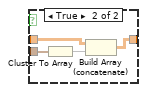
[diagram p17: hidden frame]
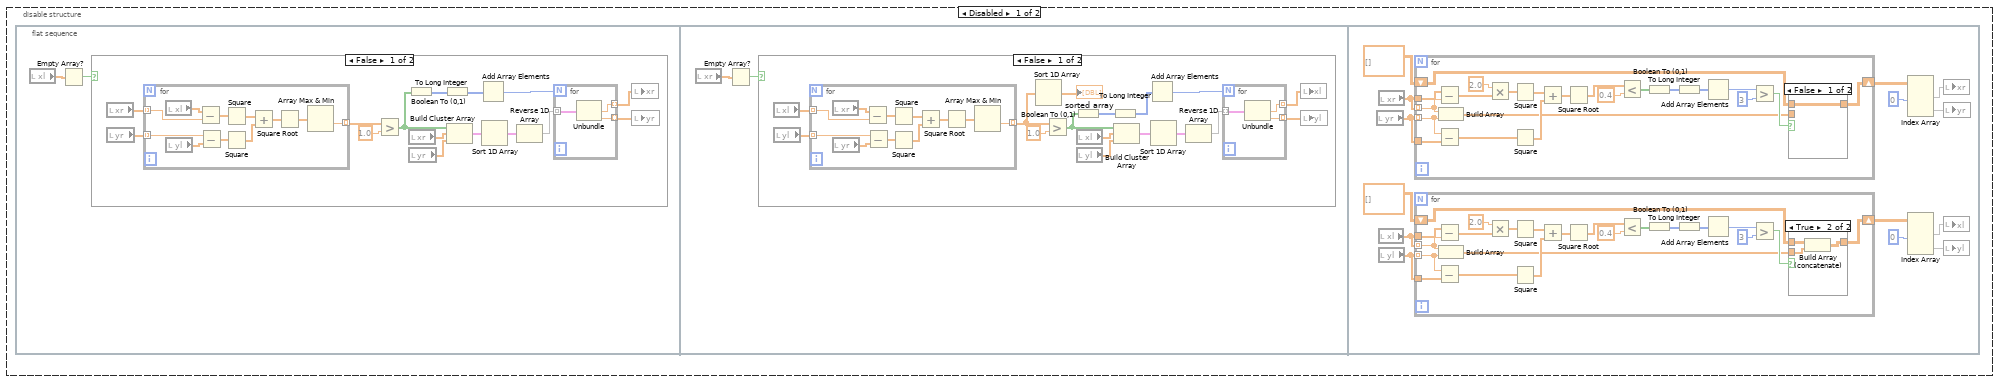
[diagram p19: hidden frame]
diagram:
  n1 = case shown="True" "update" {
    frame False {
      n2 = global write "G_SEN.vi" "laser x shift"(0.0 ("laser x shift")) -> ()
      n3 = global write "G_SEN.vi" "laser y shift"(0.0 ("laser y shift")) -> ()
    }
    frame True {
      n4 = flat-sequence {
        frame #0 {
          n5 = First Call?() -> (First Call?: T/F=w4:bool)
          n6 = case shown="True" w4 {
            frame False {
            }
            frame True {
              n7 = flat-sequence {
                frame #0 {
                  w20 = 3.141592653589793
                  n8 = global read "G_ALL.vi" "CARSPEC"() -> (w38:T1)
                  n9 = Negate(x=w20) -> (-x=w21:dbl)
                  n10 = Unbundle By Name(w38) -> ("C_Wheel base"=w18:dbl, "turn radius"=w37:dbl, "Overall width"=w32:dbl, "C_Wheel base"=w7:dbl)
                  n11 = call-poly <vilib>:"Ramp Pattern.vi"("start"=w21, "end"=w20, "delta"=0.01) -> ("Ramp Pattern"=w16:dbl[])  [unwired: 6 in, 2 out]
                  n12 = Divide(x=w18, y=w37) -> (x/y=w36:dbl)
                  n13 = Add(x=w7, y=1.0) -> (x+y=w5:dbl)
                  "af" <- w5
                  n14 = Multiply(x=w32, y=0.5) -> (x*y=w17:dbl)
                  n15 = disable-structure shown="Enabled" {
                    disable-tunnel: w17 -> [w43 w44]
                    disable-tunnel: [w40 w44] -> w8
                    frame Disabled {
                      n16 = Add(x=w43, y=0.1) -> (x+y=w41:dbl)
                      n17 = Max & Min(x=w41, y=0.8) -> (min(x,y)=w40:dbl)  [unwired: 1 out]
                    }
                    frame Enabled {
                    }
                  }
                  "gap" <- w8
                  n18 = Inverse Tangent(1:w36) -> (0:w35:dbl)
                  n19 = Negate(x=3.141592653589793) -> (-x=w13:dbl)
                  n20 = Build Array (concatenate)(w16, w13) -> (→"theta":dbl[])
                  n21 = Negate(x=w35) -> (-x=w9:dbl)
                  n22 = call-poly <vilib>:"Ramp Pattern.vi"("start"=w9, "end"=w35, "delta"=0.025) -> ("Ramp Pattern"=w33:dbl[])  [unwired: 6 in, 2 out]
                  n23 = Square(x=w5) -> (x^2=w26:dbl)
                  n24 = Tangent(1:w33) -> (0:w30:dbl[])
                  n25 = Divide(x=w18, y=w30) -> (x/y=w12:dbl[])
                  "r" <- w12
                  n26 = Sign(1:w30) -> (0:w29:dbl[])
                  n27 = Multiply(x=w29, y=w8) -> (x*y=w28:dbl[])
                  n28 = Subtract(x=w12, y=w28) -> (x-y=→"rin":dbl[])
                  n29 = Add(x=w12, y=w28) -> (x+y=w24:dbl[])
                  n30 = Square(x=w24) -> (x^2=w27:dbl[])
                  n31 = Sign(1:w24) -> (0:w22:dbl[])
                  n32 = Add(x=w27, y=w26) -> (x+y=w25:dbl[])
                  n33 = Square Root(x=w25) -> (sqrt(x)=w23:dbl[])
                  n34 = Multiply(x=w22, y=w23) -> (x*y=→"rout":dbl[])
                }
                frame #1 {
                  w50 = 0.0 ("element")
                  n35 = disable-structure shown="Enabled" {
                    frame Disabled {
                      n36 = local write "d_safe"(0.6 ("d_safe")) -> ()
                    }
                    frame Enabled {
                    }
                  }
                  n37 = local read "gap"() -> (w57:dbl)
                  n38 = local read "af"() -> (w52:dbl)
                  n39 = Negate(x=w57) -> (-x=w55:dbl)
                  n40 = Build Array(0.0 ("element"), w52, w52, w50, w50) -> (→"y_car":dbl[])
                  n41 = local read "gap"() -> (w56:dbl)
                  n42 = local read "gap"() -> (w54:dbl)
                  n43 = call-poly <vilib>:"Ramp Pattern.vi"("start"=-1.0, "end"=6.0, "delta"=0.25) -> ("Ramp Pattern"=→"y_ramp":dbl[])  [unwired: 6 in, 2 out]
                  n44 = Build Array(w56, w56, w55, w55, w54) -> (→"x_car":dbl[])
                }
              }
            }
          }
        }
        frame #1 {
          n45 = disable-structure shown="Enabled" {
            disable-tunnel: [w97 _] -> w61
            frame Enabled {
              n46 = global read "G_ALL.vi" "dist"() -> (w104:dbl[])
              n47 = Threshold 1D Array(2:-4.0 ("threshold y"), 3:w104) -> (0:w102:dbl)  [unwired: 1 in]
              n48 = global read "G_ALL.vi" "mission num"() -> (w99:i32)
              n49 = Round Toward -Infinity(1:w102) -> (0:w101:dbl)
              n50 = To Long Integer(number=w101) -> (32bit integer=w96:i32)
              n51 = Equal?(x=w99, y=6) -> (x = y?=w98:bool)
              n52 = Select(t=0, s=w98, f=w96) -> (s? t:f=w97:i32)
            }
            frame Disabled {
            }
          }
          n53 = global read "G_ALL.vi" "Steering coeff"() -> (w69:dbl[])
          n54 = Index Array(array=w69, index=0) -> (element=→"R0":dbl)
          n55 = global read "G_ALL.vi" "map_track 2"() -> (w63:dbl[][])
          n56 = global read "G_ALL.vi" "v origin 2"() -> (w65:dbl[])
          n57 = Array Subset(array=w63, index (row)=w61) -> (w62:dbl[][])  [unwired: 3 in]
          n58 = Empty Array?(array=w62) -> (empty?=w66:bool)
          n59 = Array Subset(array=w65, index=w61) -> (w64:dbl[])  [unwired: 1 in]
          n60 = case shown="False" w66 {
            tunnel: [w137 w156] -> w71
            tunnel: [w135 w147] -> w60
            tunnel: [w136 w155] -> w70
            tunnel: w62 -> [w134 _]
            tunnel: w64 -> [w105 _]
            frame False {
              n61 = Array Size(array=w134) -> (size(s)=w131:i32[])
              n62 = Index Array(array=w105, index=0) -> (element=w112:dbl)
              "element" <- w112
              n63 = Index Array(array=w131, index=0) -> (element=w129:i32)
              n64 = Decrement(x=w129) -> (x-1=w121:i32)
              n65 = Array Subset(array=w134, index (row)=1 ("index")) -> (w127:dbl[][])  [unwired: 3 in]
              n66 = Less Than 0?(x=w112) -> (x < 0?=w110:bool)
              n67 = Decrement(x=w121) -> (x-1=w120:i32)
              n68 = Array Subset(array=w134, index (row)=0 ("index"), length (row)=w121) -> (w128:dbl[][])  [unwired: 2 in]
              n69 = Subtract(x=w127, y=w128) -> (x-y=w126:dbl[][])
              n70 = Select(t=3.141592653589793, s=w110, f=0.0) -> (s? t:f=w108:dbl)
              n71 = Index Array(array=w126, index (col) #1=0 ("disabled index (col)"), index (col) #2=1 ("index (col)")) -> (element #1=w123:dbl[], element #2=w122:dbl[])  [unwired: 2 in]
              n72 = Inverse Tangent (2 Input)(1:w122, 2:w123) -> (0:w118:dbl[])
              n73 = Index Array(array=w118, index=w120) -> (element=w114:dbl)
              n74 = Delete From Array(array=w118, index=0) -> (deleted portion=w111:dbl, array with subset deleted=w116:dbl[])  [unwired: 1 in]
              n75 = call "headingoperater.vi"("h1"=w108, "h2"=w111) -> ("h2-h1"=w107:dbl)  [unwired: 8 in, 1 out]
              n76 = for {
                tunnel: w116 -> [w140] mode=indexing
                shift-right: [w141] -> _
                shift-left: w107 -> [w139]
                tunnel: [w141] -> w115 mode=indexing
                n77 = call "headingoperater.vi"("h1"=w139, "h2"=w140) -> ("h2-h1"=w138:dbl)  [unwired: 8 in, 1 out]
                n78 = call "headingoperater.vi"("h1"=3.141592653589793, "h2"=w140) -> ("h2-h1"=w143:dbl)  [unwired: 8 in, 1 out]
                n79 = Absolute Value(x=w138) -> (abs(x)=w146:dbl)
                n80 = Less?(x=w146, y=1.5707963267948966) -> (x < y?=w144:bool)
                n81 = Select(t=w140, s=w144, f=w143) -> (s? t:f=w141:dbl)
              }
              n82 = Build Array (concatenate)(w107, w115, w114) -> (w135:dbl[])
              n83 = Index Array(array=w134, index (col) #1=0 ("disabled index (col)")) -> (element #1=w137:dbl[], element #2=w136:dbl[])  [unwired: 3 in]
            }
            frame True {
              n84 = global read "G_ALL.vi" "Steering coeff"() -> (w148:dbl[])
              n85 = Array Subset(array=w148, index=1) -> (w150:dbl[])  [unwired: 1 in]
              n86 = call-poly <vilib>:"nth Derivative of Polynomial.vi"("order"=1, "P(x)"=w150) -> ("Nth Derivative of P(x)"=w151:dbl[])  [unwired: 8 in, 1 out]
              n87 = for {
                N: 49 -> [_]
                shift-right: [w157] -> _
                shift-left: -4.0 -> [w158]
                tunnel: w151 -> [w166]
                tunnel: w150 -> [w162]
                tunnel: [w161] -> w156 mode=indexing
                tunnel: [w158] -> w155 mode=indexing
                tunnel: [w160] -> w147 mode=indexing
                n88 = call-poly <vilib>:"Polynomial Evaluation.vi"("P(x)"=w166, "a"=w158) -> ("P(a)"=w165:dbl)  [unwired: 1 out]
                n89 = call-poly <vilib>:"Polynomial Evaluation.vi"("P(x)"=w162, "a"=w158) -> ("P(a)"=w161:dbl)  [unwired: 1 out]
                n90 = Inverse Tangent(1:w165) -> (0:w160:dbl)
                n91 = Cosine(x=w160) -> (cos(x)=w164:dbl)
                n92 = Multiply(x=w164, y=0.25) -> (x*y=w159:dbl)
                n93 = Add(x=w158, y=w159) -> (x+y=w157:dbl)
              }
            }
          }
          "y_path" <- w70
          "x_path" <- w71
          n94 = disable-structure shown="Enabled" {
            disable-tunnel: w60 -> [w73 w80 w82]
            disable-tunnel: [w72 w80 w83] -> w59
            frame Disabled {
              w76 = 0.0
              n95 = Array Size(array=w73) -> (size(s)=w75:i32)
              n96 = Add(x=w73, y=w76) -> (x+y=w74:dbl[])
              n97 = Multiply(x=w76, y=w75) -> (x*y=w77:dbl)
              n98 = Add(x=w77, y=1.0) -> (x+y=w79:dbl)
              n99 = Divide(x=w74, y=w79) -> (x/y=w72:dbl[])
            }
            frame Enabled {
            }
            frame Disabled {
              n100 = Index Array(array=w82) -> (element=w84:dbl)  [unwired: 1 in]
              n101 = Array Subset(array=w82, index=1) -> (w86:dbl[])  [unwired: 1 in]
              n102 = for {
                tunnel: w86 -> [w94] mode=indexing
                tunnel: 0.8 ("LPFGAIN") -> [w93]
                shift-right: [w88] -> _
                shift-left: w84 -> [w89]
                tunnel: [w88] -> w85 mode=indexing
                n103 = Multiply(x=w94, y=w93) -> (x*y=w91:dbl)
                n104 = Decrement(x=w93) -> (x-1=w92:dbl)
                n105 = Multiply(x=w92, y=w89) -> (x*y=w90:dbl)
                n106 = Subtract(x=w91, y=w90) -> (x-y=w88:dbl)
              }
              n107 = Build Array (concatenate)(w84, w85) -> (w83:dbl[])
            }
          }
          "h_path" <- w59
        }
        frame #2 {
          n108 = local read "gap"() -> (w182:dbl)
          n109 = local read "h_path"() -> (w183:dbl[])
          n110 = local read "h_path"() -> (w172:dbl[])
          n111 = Negate(x=w182) -> (-x=w181:dbl)
          n112 = local read "y_path"() -> (w184:dbl[])
          n113 = local read "x_path"() -> (w185:dbl[])
          n114 = local read "y_path"() -> (w171:dbl[])
          n115 = local read "x_path"() -> (w170:dbl[])
          n116 = local read "gap"() -> (w167:dbl)
          n117 = local read "af"() -> (w169:dbl)
          n118 = local read "af"() -> (w168:dbl)
          n119 = for {
            tunnel: w185 -> [w205] mode=indexing
            tunnel: w184 -> [w204] mode=indexing
            tunnel: w183 -> [w206] mode=indexing
            tunnel: [w209] -> w180 mode=indexing
            tunnel: [w208] -> w179 mode=indexing
            tunnel: w181 -> [w203]
            tunnel: [w201] -> w178 mode=indexing
            tunnel: [w200] -> w177 mode=indexing
            tunnel: w169 -> [w198]
            n120 = call "rotm_siso.vi"("angle[rad]"=w206, "reverse"=TRUE, "y0"=w205, "x0"=w204, "y"=w203, "x"=0.0) -> ("y'"=w200:dbl, "x'"=w201:dbl)  [unwired: 4 in]
            n121 = call "rotm_siso.vi"("angle[rad]"=w206, "reverse"=TRUE, "y0"=w205, "x0"=w204, "y"=w203, "x"=w198) -> ("y'"=w208:dbl, "x'"=w209:dbl)  [unwired: 4 in]
          }
          "x_lf" <- w179
          "y_lf" <- w180
          "y_lr" <- w178
          "x_lr" <- w177
          n122 = for {
            tunnel: w170 -> [w193] mode=indexing
            tunnel: w171 -> [w192] mode=indexing
            tunnel: w172 -> [w194] mode=indexing
            tunnel: [w197] -> w173 mode=indexing
            tunnel: [w196] -> w174 mode=indexing
            tunnel: [w190] -> w175 mode=indexing
            tunnel: [w189] -> w176 mode=indexing
            tunnel: w168 -> [w187]
            tunnel: w167 -> [w186]
            n123 = call "rotm_siso.vi"("angle[rad]"=w194, "reverse"=TRUE, "y0"=w193, "x0"=w192, "y"=w186, "x"=0.0) -> ("y'"=w189:dbl, "x'"=w190:dbl)  [unwired: 4 in]
            n124 = call "rotm_siso.vi"("angle[rad]"=w194, "reverse"=TRUE, "y0"=w193, "x0"=w192, "y"=w186, "x"=w187) -> ("y'"=w196:dbl, "x'"=w197:dbl)  [unwired: 4 in]
          }
          "x_rf" <- w174
          "y_rf" <- w173
          "y_rr" <- w175
          "x_rr" <- w176
        }
        frame #3 {
          n125 = local read "y_path"() -> (w249:dbl[])
          n126 = local read "y_lf"() -> (w216:dbl[])
          n127 = local read "x_rf"() -> (w212:dbl[])
          n128 = local read "y_rf"() -> (w213:dbl[])
          n129 = local read "x_lf"() -> (w217:dbl[])
          n130 = for {
            tunnel: w217 -> [w299] mode=indexing
            tunnel: w216 -> [w298] mode=indexing
            tunnel: [w288] -> w215 mode=indexing
            n131 = local read "x_path"() -> (w300:dbl[])
            n132 = local read "y_path"() -> (w297:dbl[])
            n133 = Subtract(x=w300, y=w299) -> (x-y=w292:dbl[])
            n134 = Subtract(x=w298, y=w297) -> (x-y=w291:dbl[])
            n135 = Square(x=w292) -> (x^2=w293:dbl[])
            n136 = Square(x=w291) -> (x^2=w294:dbl[])
            n137 = Add(x=w293, y=w294) -> (x+y=w295:dbl[])
            n138 = Square Root(x=w295) -> (sqrt(x)=w296:dbl[])
            n139 = local read "h_path"() -> (w290:dbl[])
            n140 = Array Max & Min(array=w296) -> (min index (indices)=w289:i32)  [unwired: 3 out]
            n141 = Index Array(array=w290, index=w289) -> (element=w288:dbl)
          }
          "h_lf" <- w215
          n142 = for {
            tunnel: w212 -> [w286] mode=indexing
            tunnel: w213 -> [w285] mode=indexing
            tunnel: [w275] -> w214 mode=indexing
            n143 = local read "x_path"() -> (w287:dbl[])
            n144 = local read "y_path"() -> (w284:dbl[])
            n145 = Subtract(x=w287, y=w286) -> (x-y=w279:dbl[])
            n146 = Subtract(x=w285, y=w284) -> (x-y=w278:dbl[])
            n147 = Square(x=w279) -> (x^2=w280:dbl[])
            n148 = Square(x=w278) -> (x^2=w281:dbl[])
            n149 = Add(x=w280, y=w281) -> (x+y=w282:dbl[])
            n150 = Square Root(x=w282) -> (sqrt(x)=w283:dbl[])
            n151 = local read "h_path"() -> (w277:dbl[])
            n152 = Array Max & Min(array=w283) -> (min index (indices)=w276:i32)  [unwired: 3 out]
            n153 = Index Array(array=w277, index=w276) -> (element=w275:dbl)
          }
          "h_rf" <- w214
          n154 = local read "x_path"() -> (w250:dbl[])
          n155 = Array Size(array=w249) -> (size(s)=w247:i32)
          n156 = global read "G_ALL.vi" "mission num"() -> (w210:i32)
          n157 = Build Array(w250, w249) -> (w248:dbl[][])
          n158 = Decrement(x=w247) -> (x-1=w246:i32)
          n159 = case shown="60" w210 {
            tunnel: [w253 _] -> w211
            frame 0, Default {
              n160 = local read "gap"() -> (w270:dbl)
              n161 = local read "y_lf"() -> (w272:dbl[])
              n162 = local read "y_rf"() -> (w273:dbl[])
              n163 = Negate(x=w270) -> (-x=w269:dbl)
              n164 = local read "af"() -> (w268:dbl)
              n165 = local read "gap"() -> (w255:dbl)
              n166 = local read "af"() -> (w254:dbl)
              n167 = local read "x_lf"() -> (w271:dbl[])
              n168 = local read "x_rf"() -> (w274:dbl[])
              n169 = Subtract(x=w268, y=w272) -> (x-y=w258:dbl[])
              n170 = Subtract(x=w254, y=w273) -> (x-y=w256:dbl[])
              n171 = Subtract(x=w271, y=w269) -> (x-y=w259:dbl[])
              n172 = Subtract(x=w274, y=w255) -> (x-y=w257:dbl[])
              n173 = Square(x=w259) -> (x^2=w260:dbl[])
              n174 = Square(x=w258) -> (x^2=w261:dbl[])
              n175 = Square(x=w257) -> (x^2=w267:dbl[])
              n176 = Square(x=w256) -> (x^2=w266:dbl[])
              n177 = Add(x=w260, y=w261) -> (x+y=w262:dbl[])
              n178 = Add(x=w267, y=w266) -> (x+y=w265:dbl[])
              n179 = Square Root(x=w262) -> (sqrt(x)=w263:dbl[])
              n180 = Square Root(x=w265) -> (sqrt(x)=w264:dbl[])
              n181 = Array Max & Min(array=w263) -> (min index (indices)=w252:i32)  [unwired: 3 out]
              n182 = Array Max & Min(array=w264) -> (min index (indices)=w251:i32)  [unwired: 3 out]
              n183 = Max & Min(x=w252, y=w251) -> (min(x,y)=w253:i32)  [unwired: 1 out]
            }
            frame 60 {
            }
          }
          "idxfront" <- w211
          n184 = Index Array(array=w248, index (col)=w246) -> (element=w221:dbl[])  [unwired: 1 in]
          n185 = Index Array(array=w221, index #1=0 ("index")) -> (element #1=w244:dbl, element #2=w242:dbl)  [unwired: 1 in]
          n186 = Index Array(array=w221, index #1=0 ("index")) -> (element #1=w223:dbl, element #2=w225:dbl)  [unwired: 1 in]
          n187 = local read "y_lf"() -> (w241:dbl[])
          n188 = local read "x_rf"() -> (w224:dbl[])
          n189 = local read "y_rf"() -> (w226:dbl[])
          n190 = local read "x_lf"() -> (w243:dbl[])
          n191 = Subtract(x=w243, y=w244) -> (x-y=w239:dbl[])
          n192 = Subtract(x=w242, y=w241) -> (x-y=w240:dbl[])
          n193 = Subtract(x=w224, y=w223) -> (x-y=w228:dbl[])
          n194 = Subtract(x=w225, y=w226) -> (x-y=w227:dbl[])
          n195 = Square(x=w239) -> (x^2=w238:dbl[])
          n196 = Square(x=w240) -> (x^2=w237:dbl[])
          n197 = Square(x=w228) -> (x^2=w229:dbl[])
          n198 = Square(x=w227) -> (x^2=w230:dbl[])
          n199 = Add(x=w238, y=w237) -> (x+y=w236:dbl[])
          n200 = Add(x=w229, y=w230) -> (x+y=w231:dbl[])
          n201 = Square Root(x=w236) -> (sqrt(x)=w235:dbl[])
          n202 = Square Root(x=w231) -> (sqrt(x)=w232:dbl[])
          n203 = Array Max & Min(array=w235) -> (min index (indices)=w234:i32)  [unwired: 3 out]
          n204 = Array Max & Min(array=w232) -> (min index (indices)=w233:i32)  [unwired: 3 out]
          n205 = Increment(x=w234) -> (x+1=w220:i32)
          n206 = Increment(x=w233) -> (x+1=w219:i32)
          n207 = Max & Min(x=w220, y=w219) -> (max(x,y)=→"size limit":i32)  [unwired: 1 out]
        }
        frame #4 {
          n208 = disable-structure shown="Enabled" {
            disable-tunnel: [w308 w312] -> w305
            disable-tunnel: [w307 w314] -> w304
            disable-tunnel: [w306 w310] -> w301
            frame Disabled {
              n209 = global read "G_LCM.vi" "VISION_LANE_PT"() -> (w309:T2)
              n210 = Unbundle By Name(w309) -> ("point_flag"=w306:i32[], "x"=w308:dbl[], "y"=w307:dbl[])
            }
            frame Enabled {
              n211 = global read "G_SEN.vi" "SICK_laser"() -> (w315:dbl[][])
              n212 = Index Array(array=w315, index (col) #1=0 ("disabled index (col)"), index (col) #2=1 ("index (col)")) -> (element #1=w312:dbl[], element #2=w314:dbl[])  [unwired: 2 in]
              n213 = To Long Integer(number=w312) -> (32bit integer=w311:i32[])
              n214 = Multiply(x=0, y=w311) -> (x*y=w310:i32[])
            }
          }
          n215 = disable-structure shown="Enabled" {
            disable-tunnel: w305 -> [w334 w345 w361]
            disable-tunnel: [w332 w344 w359] -> w302
            disable-tunnel: [w331 w345 w361] -> w303
            disable-tunnel: w304 -> [w328 w344 w359]
            disable-tunnel: w301 -> [_ _ w360]
            frame Disabled {
              n216 = disable-structure shown="Enabled" {
                disable-tunnel: w334 -> [w337 w338]
                disable-tunnel: [w336 w338] -> w335
                frame Disabled {
                  n217 = Negate(x=w337) -> (-x=w336:dbl[])
                }
                frame Enabled {
                }
              }
              n218 = In Range and Coerce(upper limit=6.0 ("delta"), x=w328, lower limit=-5.0) -> (In Range?=w326:bool[])  [unwired: 1 out]
              n219 = Build Cluster Array(w326, w335, w328) -> (w324:T3)
              n220 = Sort 1D Array(array=w324) -> (sorted array=w325:T3)
              n221 = Reverse 1D Array(array=w325) -> (reversed array=w321:T3)
              n222 = for {
                tunnel: w321 -> [w342] mode=indexing
                tunnel: [w341] -> w319 mode=indexing
                tunnel: [w340] -> w318 mode=indexing
                tunnel: [w339] -> w329 mode=indexing
                n223 = Unbundle(w342) -> ("delta"=w339:bool, "element"=w341:dbl, "element"=w340:dbl)
              }
              n224 = Boolean To (0,1)(Boolean=w329) -> (0, 1=w322:i16[])
              n225 = Add Array Elements(numeric array=w322) -> (sum=w330:i16)
              n226 = Delete From Array(array=w319, length=w330, index=0) -> (deleted portion=w331:dbl[])  [unwired: 1 out]
              n227 = Delete From Array(array=w318, length=w330, index=0) -> (deleted portion=w332:dbl[])  [unwired: 1 out]
            }
            frame Enabled {
              w343 = dbl[] [] ("yl")
              n228 = local write "yl"(w343) -> ()
              n229 = local write "yr"(w343) -> ()
              n230 = local write "xl"(w343) -> ()
              n231 = local write "xr"(w343) -> ()
            }
            frame Disabled {
              n232 = global read "G_ALL.vi" "mission num"() -> (w347:i32)
              n233 = case shown="2, 4, 6" w347 {
                tunnel: [10.0 10.0] -> w346
                frame 0, Default {
                }
                frame 2, 4, 6 {
                }
              }
              n234 = In Range and Coerce(upper limit=w346, x=w359, lower limit=-6.0) -> (In Range?=w351:bool[])  [unwired: 1 out]
              n235 = Boolean To (0,1)(Boolean=w351) -> (0, 1=w350:i16[])
              n236 = Build Cluster Array(w351, w360, w361, w359) -> (w357:T4)
              n237 = To Long Integer(number=w350) -> (32bit integer=w349:i32[])
              n238 = Sort 1D Array(array=w357) -> (sorted array=w356:T4)
              n239 = Add Array Elements(numeric array=w349) -> (sum=w348:i32)
              n240 = Reverse 1D Array(array=w356) -> (reversed array=w355:T4)
              n241 = for {
                N: w348 -> [_]
                tunnel: w355 -> [w461] mode=indexing
                tunnel: [w460] -> w354 mode=indexing
                tunnel: [w459] -> w353 mode=indexing
                tunnel: [w458] -> w352 mode=indexing
                n242 = Unbundle(w461) -> (w460:i32, "element"=w459:dbl, "element"=w458:dbl)  [unwired: 1 out]
              }
              n243 = Build Cluster Array(w354, w353, w352) -> (w393:cluster{i32, "element":dbl, "element":dbl}[])
              n244 = Sort 1D Array(array=w393) -> (sorted array=w392:cluster{i32, "element":dbl, "element":dbl}[])
              n245 = for {
                tunnel: w392 -> [w465] mode=indexing
                tunnel: [w464] -> w391 mode=indexing
                tunnel: [w462] -> w390 mode=indexing
                tunnel: [w463] -> w380 mode=indexing
                n246 = Unbundle(w465) -> (w463:i32, "element"=w464:dbl, "element"=w462:dbl)
              }
              n247 = Build Array(w391, w390) -> (w389:dbl[][])
              n248 = Not Equal?(x=w380, y=1) -> (x != y?=w378:bool[])
              n249 = Equal?(x=w380, y=-1) -> (x = y?=w384:bool[])
              n250 = Boolean To (0,1)(Boolean=w384) -> (0, 1=w383:i16[])
              n251 = Boolean To (0,1)(Boolean=w378) -> (0, 1=w377:i16[])
              n252 = To Long Integer(number=w383) -> (32bit integer=w382:i32[])
              n253 = To Long Integer(number=w377) -> (32bit integer=w376:i32[])
              n254 = Add Array Elements(numeric array=w382) -> (sum=w381:i32)
              n255 = Add Array Elements(numeric array=w376) -> (sum=w374:i32)
              n256 = Transpose 2D Array(2D array=w389) -> (transposed array=w375:dbl[][])
              n257 = Array Subset(array=w375, index (row)=w374) -> (w372:dbl[][])  [unwired: 3 in]
              n258 = Array Subset(array=w375, index (row)=0 ("index"), length (row)=w381) -> (w387:dbl[][])  [unwired: 2 in]
              n259 = Index Array(array=w387, index (col) #1=0 ("disabled index (col)")) -> (element #1=w366:dbl[], element #2=w364:dbl[])  [unwired: 3 in]
              n260 = Index Array(array=w372, index (col) #1=0 ("disabled index (col)")) -> (element #1=w371:dbl[], element #2=w369:dbl[])  [unwired: 3 in]
              n261 = disable-structure shown="Enabled" {
                disable-tunnel: w371 -> [w429 w455]
                disable-tunnel: [w428 w455] -> w370
                disable-tunnel: w369 -> [w427 w454]
                disable-tunnel: [w426 w454] -> w367
                disable-tunnel: w366 -> [w425 w457]
                disable-tunnel: [w424 w457] -> w365
                disable-tunnel: w364 -> [w423 w456]
                disable-tunnel: [w422 w456] -> w362
                frame Enabled {
                  w408 = 10.0
                  w421 = 10.0
                  n262 = Multiply(x=w425, y=w421) -> (x*y=w420:dbl[])
                  n263 = Multiply(x=w421, y=w423) -> (x*y=w419:dbl[])
                  n264 = Multiply(x=w429, y=w408) -> (x*y=w407:dbl[])
                  n265 = Multiply(x=w408, y=w427) -> (x*y=w406:dbl[])
                  n266 = Round To Nearest(number=w420) -> (nearest integer value=w417:dbl[])
                  n267 = Round To Nearest(number=w419) -> (nearest integer value=w418:dbl[])
                  n268 = Round To Nearest(number=w407) -> (nearest integer value=w404:dbl[])
                  n269 = Round To Nearest(number=w406) -> (nearest integer value=w405:dbl[])
                  n270 = Build Cluster Array(w417, w418) -> (w416:cluster{dbl, dbl}[])
                  n271 = Build Cluster Array(w404, w405) -> (w403:cluster{dbl, dbl}[])
                  n272 = Sort 1D Array(array=w416) -> (sorted array=w415:cluster{dbl, dbl}[])
                  n273 = Sort 1D Array(array=w403) -> (sorted array=w402:cluster{dbl, dbl}[])
                  n274 = for {
                    tunnel: w415 -> [w430] mode=indexing
                    shift-right: [w430] -> _
                    shift-left: cluster{dbl, dbl} {inf, inf} ("output cluster") -> [w436]
                    shift-right: [w432] -> w412
                    shift-left: dbl[][] [] -> [w431]
                    n275 = Not Equal?(x=w436, y=w430) -> (x != y?=w435:cluster{bool, bool})
                    n276 = Cluster To Array(cluster=w435) -> (array=w434:bool[])
                    n277 = Or Array Elements(Boolean array=w434) -> (logical OR=w433:bool)
                    n278 = case shown="True" w433 {
                      tunnel: w430 -> [_ w441]
                      tunnel: [w437 w439] -> w432
                      tunnel: w431 -> [w437 w438]
                      frame False {
                      }
                      frame True {
                        n279 = Cluster To Array(cluster=w441) -> (array=w440:dbl[])
                        n280 = Build Array (concatenate)(w438, w440) -> (w439:dbl[][])
                      }
                    }
                  }
                  n281 = for {
                    tunnel: w402 -> [w442] mode=indexing
                    shift-right: [w442] -> _
                    shift-left: cluster{dbl, dbl} {inf, inf} ("output cluster") -> [w448]
                    shift-right: [w444] -> w399
                    shift-left: dbl[][] [] -> [w443]
                    n282 = Not Equal?(x=w448, y=w442) -> (x != y?=w447:cluster{bool, bool})
                    n283 = Cluster To Array(cluster=w447) -> (array=w446:bool[])
                    n284 = Or Array Elements(Boolean array=w446) -> (logical OR=w445:bool)
                    n285 = case shown="False" w445 {
                      tunnel: w442 -> [_ w453]
                      tunnel: [w449 w451] -> w444
                      tunnel: w443 -> [w449 w450]
                      frame False {
                      }
                      frame True {
                        n286 = Cluster To Array(cluster=w453) -> (array=w452:dbl[])
                        n287 = Build Array (concatenate)(w450, w452) -> (w451:dbl[][])
                      }
                    }
                  }
                  n288 = Multiply(x=w412, y=0.1) -> (x*y=w410:dbl[][])
                  n289 = Multiply(x=w399, y=0.1) -> (x*y=w397:dbl[][])
                  n290 = Index Array(array=w410, index (col) #1=0 ("disabled index (col)")) -> (element #1=w424:dbl[], element #2=w422:dbl[])  [unwired: 3 in]
                  n291 = Index Array(array=w397, index (col) #1=0 ("disabled index (col)")) -> (element #1=w428:dbl[], element #2=w426:dbl[])  [unwired: 3 in]
                }
                frame Disabled {
                }
              }
              "xl" <- w365
              "yl" <- w362
              "xr" <- w370
              "yr" <- w367
              n292 = Array Size(array=w362) -> (size(s)=→"size(s) 4":i32)
              n293 = Array Size(array=w367) -> (size(s)=→"size(s) 3":i32)
            }
          }
          "x" <- w303
          "y" <- w302
        }
        frame #5 {
          n294 = disable-structure shown="Enabled" {
            frame Disabled {
              n295 = flat-sequence {
                frame #0 {
                  n296 = local read "xl"() -> (w467:dbl[])
                  n297 = Empty Array?(array=w467) -> (empty?=w466:bool)
                  n298 = case shown="False" w466 {
                    frame False {
                      n299 = local read "xr"() -> (w482:dbl[])
                      n300 = local read "yr"() -> (w481:dbl[])
                      n301 = for {
                        tunnel: w482 -> [w495] mode=indexing
                        tunnel: w481 -> [w493] mode=indexing
                        tunnel: [w486] -> w480 mode=indexing
                        n302 = local read "xl"() -> (w496:dbl[])
                        n303 = local read "yl"() -> (w494:dbl[])
                        n304 = Subtract(x=w496, y=w495) -> (x-y=w492:dbl[])
                        n305 = Subtract(x=w493, y=w494) -> (x-y=w491:dbl[])
                        n306 = Square(x=w492) -> (x^2=w490:dbl[])
                        n307 = Square(x=w491) -> (x^2=w489:dbl[])
                        n308 = Add(x=w490, y=w489) -> (x+y=w488:dbl[])
                        n309 = Square Root(x=w488) -> (sqrt(x)=w487:dbl[])
                        n310 = Array Max & Min(array=w487) -> (min value=w486:dbl)  [unwired: 3 out]
                      }
                      n311 = Greater?(x=w480, y=1.0) -> (0:w472:bool[])
                      n312 = Boolean To (0,1)(Boolean=w472) -> (0, 1=w471:i16[])
                      n313 = local read "xr"() -> (w476:dbl[])
                      n314 = local read "yr"() -> (w475:dbl[])
                      n315 = To Long Integer(number=w471) -> (32bit integer=w470:i32[])
                      n316 = Build Cluster Array(w472, w476, w475) -> (w474:T5)
                      n317 = Add Array Elements(numeric array=w470) -> (sum=w469:i32)
                      n318 = Sort 1D Array(array=w474) -> (sorted array=w473:T5)
                      n319 = Reverse 1D Array(array=w473) -> (reversed array=w468:T5)
                      n320 = for {
                        N: w469 -> [_]
                        tunnel: w468 -> [w485] mode=indexing
                        tunnel: [w484] -> w479 mode=indexing
                        tunnel: [w483] -> w478 mode=indexing
                        n321 = Unbundle(w485) -> ("Rotational position"=w484:dbl, "Rotational position"=w483:dbl)  [unwired: 1 out]
                      }
                      n322 = local write "xr"(w479) -> ()
                      n323 = local write "yr"(w478) -> ()
                    }
                    frame True {
                    }
                  }
                }
                frame #1 {
                  n324 = local read "xr"() -> (w498:dbl[])
                  n325 = Empty Array?(array=w498) -> (empty?=w497:bool)
                  n326 = case shown="False" w497 {
                    frame False {
                      n327 = local read "xl"() -> (w514:dbl[])
                      n328 = local read "yl"() -> (w513:dbl[])
                      n329 = for {
                        tunnel: w514 -> [w527] mode=indexing
                        tunnel: w513 -> [w525] mode=indexing
                        tunnel: [w518] -> w500 mode=indexing
                        n330 = local read "xr"() -> (w528:dbl[])
                        n331 = local read "yr"() -> (w526:dbl[])
                        n332 = Subtract(x=w528, y=w527) -> (x-y=w524:dbl[])
                        n333 = Subtract(x=w525, y=w526) -> (x-y=w523:dbl[])
                        n334 = Square(x=w524) -> (x^2=w522:dbl[])
                        n335 = Square(x=w523) -> (x^2=w521:dbl[])
                        n336 = Add(x=w522, y=w521) -> (x+y=w520:dbl[])
                        n337 = Square Root(x=w520) -> (sqrt(x)=w519:dbl[])
                        n338 = Array Max & Min(array=w519) -> (min value=w518:dbl)  [unwired: 3 out]
                      }
                      n339 = Sort 1D Array(array=w500) -> (sorted array=→"sorted array":dbl[])
                      n340 = Greater?(x=w500, y=1.0) -> (0:w507:bool[])
                      n341 = Boolean To (0,1)(Boolean=w507) -> (0, 1=w506:i16[])
                      n342 = local read "xl"() -> (w511:dbl[])
                      n343 = local read "yl"() -> (w510:dbl[])
                      n344 = To Long Integer(number=w506) -> (32bit integer=w505:i32[])
                      n345 = Build Cluster Array(w507, w511, w510) -> (w509:T5)
                      n346 = Add Array Elements(numeric array=w505) -> (sum=w504:i32)
                      n347 = Sort 1D Array(array=w509) -> (sorted array=w508:T5)
                      n348 = Reverse 1D Array(array=w508) -> (reversed array=w503:T5)
                      n349 = for {
                        N: w504 -> [_]
                        tunnel: w503 -> [w517] mode=indexing
                        tunnel: [w516] -> w501 mode=indexing
                        tunnel: [w515] -> w502 mode=indexing
                        n350 = Unbundle(w517) -> ("Rotational position"=w516:dbl, "Rotational position"=w515:dbl)  [unwired: 1 out]
                      }
                      n351 = local write "xl"(w501) -> ()
                      n352 = local write "yl"(w502) -> ()
                    }
                    frame True {
                    }
                  }
                }
                frame #2 {
                  n353 = local read "yr"() -> (w530:dbl[])
                  n354 = local read "xr"() -> (w529:dbl[])
                  n355 = local read "xl"() -> (w542:dbl[])
                  n356 = local read "yl"() -> (w541:dbl[])
                  n357 = for {
                    tunnel: w529 -> [w550] mode=indexing
                    tunnel: w530 -> [w549] mode=indexing
                    tunnel: w529 -> [w555]
                    tunnel: w530 -> [w554]
                    shift-right: [w547] -> w532
                    shift-left: dbl[][] [] -> [w546]
                    n358 = Subtract(x=w555, y=w550) -> (x-y=w544:dbl[])
                    n359 = Subtract(x=w549, y=w554) -> (x-y=w564:dbl[])
                    n360 = Build Array(w550, w549) -> (w548:dbl[])
                    n361 = Multiply(x=2.0, y=w544) -> (x*y=w543:dbl[])
                    n362 = Square(x=w543) -> (x^2=w563:dbl[])
                    n363 = Square(x=w564) -> (x^2=w562:dbl[])
                    n364 = Add(x=w563, y=w562) -> (x+y=w561:dbl[])
                    n365 = Square Root(x=w561) -> (sqrt(x)=w560:dbl[])
                    n366 = Less?(x=w560, y=0.4) -> (x < y?=w558:bool[])
                    n367 = Boolean To (0,1)(Boolean=w558) -> (0, 1=w557:i16[])
                    n368 = To Long Integer(number=w557) -> (32bit integer=w556:i32[])
                    n369 = Add Array Elements(numeric array=w556) -> (sum=w553:i32)
                    n370 = Greater?(x=w553, y=3) -> (0:w551:bool)
                    n371 = case shown="False" w551 {
                      tunnel: w548 -> [_ w568]
                      tunnel: [w565 w567] -> w547
                      tunnel: w546 -> [w565 w566]
                      frame False {
                      }
                      frame True {
                        n372 = Build Array (concatenate)(w566, w568) -> (w567:dbl[][])
                      }
                    }
                  }
                  n373 = for {
                    tunnel: w542 -> [w576] mode=indexing
                    tunnel: w541 -> [w575] mode=indexing
                    tunnel: w542 -> [w581]
                    tunnel: w541 -> [w580]
                    shift-right: [w573] -> w539
                    shift-left: dbl[][] [] -> [w572]
                    n374 = Subtract(x=w581, y=w576) -> (x-y=w570:dbl[])
                    n375 = Subtract(x=w575, y=w580) -> (x-y=w590:dbl[])
                    n376 = Build Array(w576, w575) -> (w574:dbl[])
                    n377 = Multiply(x=2.0, y=w570) -> (x*y=w569:dbl[])
                    n378 = Square(x=w569) -> (x^2=w589:dbl[])
                    n379 = Square(x=w590) -> (x^2=w588:dbl[])
                    n380 = Add(x=w589, y=w588) -> (x+y=w587:dbl[])
                    n381 = Square Root(x=w587) -> (sqrt(x)=w586:dbl[])
                    n382 = Less?(x=w586, y=0.4) -> (x < y?=w584:bool[])
                    n383 = Boolean To (0,1)(Boolean=w584) -> (0, 1=w583:i16[])
                    n384 = To Long Integer(number=w583) -> (32bit integer=w582:i32[])
                    n385 = Add Array Elements(numeric array=w582) -> (sum=w579:i32)
                    n386 = Greater?(x=w579, y=3) -> (0:w577:bool)
                    n387 = case shown="True" w577 {
                      tunnel: w574 -> [_ w594]
                      tunnel: [w591 w593] -> w573
                      tunnel: w572 -> [w591 w592]
                      frame False {
                      }
                      frame True {
                        n388 = Build Array (concatenate)(w592, w594) -> (w593:dbl[][])
                      }
                    }
                  }
                  n389 = Index Array(array=w532, index (col) #1=0 ("disabled index (col)")) -> (element #1=w534:dbl[], element #2=w535:dbl[])  [unwired: 3 in]
                  n390 = Index Array(array=w539, index (col) #1=0 ("disabled index (col)")) -> (element #1=w537:dbl[], element #2=w536:dbl[])  [unwired: 3 in]
                  n391 = local write "xr"(w534) -> ()
                  n392 = local write "yr"(w535) -> ()
                  n393 = local write "xl"(w537) -> ()
                  n394 = local write "yl"(w536) -> ()
                }
              }
            }
            frame Enabled {
            }
          }
        }
        frame #6 {
          n395 = disable-structure shown="Enabled" {
            disable-tunnel: [w644 TRUE] -> w602
            frame Disabled {
              n396 = global read "G_ALL.vi" "mission num"() -> (w645:i32)
              n397 = case shown="2, 6" w645 {
                tunnel: [_ TRUE] -> w644
                frame 0, Default {
                }
                frame 2, 6 {
                }
              }
            }
            frame Enabled {
            }
          }
          n398 = local read "x"() -> (w609:dbl[])
          n399 = local read "xr"() -> (w608:dbl[])
          n400 = local read "x"() -> (w614:dbl[])
          n401 = local read "xl"() -> (w615:dbl[])
          n402 = local read "y"() -> (w604:dbl[])
          n403 = local read "yr"() -> (w605:dbl[])
          n404 = local read "y"() -> (w612:dbl[])
          n405 = local read "yl"() -> (w611:dbl[])
          n406 = Select(t=w614, s=w602, f=w615) -> (s? t:f=w613:dbl[])
          n407 = Select(t=w609, s=w602, f=w608) -> (s? t:f=w606:dbl[])
          n408 = Select(t=w612, s=w602, f=w611) -> (s? t:f=w610:dbl[])
          n409 = Select(t=w604, s=w602, f=w605) -> (s? t:f=w603:dbl[])
          n410 = Empty Array?(array=w606) -> (empty?=w607:bool)
          n411 = Empty Array?(array=w613) -> (empty?=w616:bool)
          n412 = case shown="False" w607 {
            tunnel: [w703 _] -> w640
            tunnel: [w702 _] -> w639
            tunnel: [w701 _] -> w638
            tunnel: [w700 _] -> w636
            tunnel: w606 -> [w676 _]
            tunnel: w603 -> [w675 _]
            frame False {
              n413 = local read "d_safe front"() -> (w678:dbl)
              n414 = local read "h_path"() -> (w677:dbl[])
              n415 = local read "d_safe"() -> (w662:dbl)
              n416 = local read "h_rf"() -> (w664:dbl[])
              n417 = local read "x_rf"() -> (w698:dbl[])
              n418 = local read "y_rf"() -> (w699:dbl[])
              n419 = local read "y_rr"() -> (w696:dbl[])
              n420 = local read "x_rr"() -> (w697:dbl[])
              n421 = for {
                tunnel: w676 -> [w740]
                tunnel: w675 -> [w739]
                tunnel: w699 -> [w753] mode=indexing
                tunnel: w698 -> [w737] mode=indexing
                tunnel: w677 -> [w729] mode=indexing
                tunnel: [w734] -> w666 mode=indexing
                tunnel: w678 -> [w717]
                tunnel: [w746] -> w668 mode=indexing
                tunnel: [w718] -> w654 mode=indexing
                tunnel: w697 -> [w742] mode=indexing
                tunnel: w696 -> [w741] mode=indexing
                tunnel: w664 -> [w720] mode=indexing
                tunnel: [w719] -> w663 mode=indexing
                tunnel: w662 -> [w716]
                n422 = Subtract(x=w740, y=w737) -> (x-y=w752:dbl[])
                n423 = Subtract(x=w739, y=w753) -> (x-y=w751:dbl[])
                n424 = Subtract(x=w740, y=w742) -> (x-y=w733:dbl[])
                n425 = Subtract(x=w739, y=w741) -> (x-y=w732:dbl[])
                n426 = call "headingoperater.vi"("h1"=w720, "h2"=1.5707963267948966) -> ("h2-h1"=w723:dbl)  [unwired: 8 in, 1 out]
                n427 = call "headingoperater.vi"("h1"=w729, "h2"=1.5707963267948966) -> ("h2-h1"=w728:dbl)  [unwired: 8 in, 1 out]
                n428 = Square(x=w752) -> (x^2=w749:dbl[])
                n429 = Square(x=w751) -> (x^2=w750:dbl[])
                n430 = Square(x=w732) -> (x^2=w731:dbl[])
                n431 = Square(x=w733) -> (x^2=w730:dbl[])
                n432 = Add(x=w749, y=w750) -> (x+y=w748:dbl[])
                n433 = Add(x=w731, y=w730) -> (x+y=w743:dbl[])
                n434 = call "headingoperater.vi"("h1"=1.5707963267948966, "h2"=w723) -> ("h2+h1"=w719:dbl)  [unwired: 8 in, 1 out]
                n435 = call "headingoperater.vi"("h1"=1.5707963267948966, "h2"=w728) -> ("h2+h1"=w734:dbl)  [unwired: 8 in, 1 out]
                n436 = Square Root(x=w748) -> (sqrt(x)=w747:dbl[])
                n437 = Square Root(x=w743) -> (sqrt(x)=w744:dbl[])
                n438 = Array Max & Min(array=w747) -> (min value=w736:dbl)  [unwired: 3 out]
                n439 = Array Max & Min(array=w744) -> (min value=w745:dbl)  [unwired: 3 out]
                n440 = Subtract(x=w717, y=w736) -> (x-y=w724:dbl)
                n441 = Subtract(x=w716, y=w745) -> (x-y=w725:dbl)
                n442 = Max & Min(x=w724, y=0.0) -> (max(x,y)=w746:dbl)  [unwired: 1 out]
                n443 = Max & Min(x=w725, y=0.0) -> (max(x,y)=w718:dbl)  [unwired: 1 out]
              }
              n444 = Add Array Elements(numeric array=w654) -> (sum=w680:dbl)
              n445 = Not Equal To 0?(x=w654) -> (x != 0?=w655:bool[])
              n446 = Polar To Re/Im(2:w666, 3:w654) -> (0:w692:dbl[], 1:w693:dbl[])
              n447 = disable-structure shown="Enabled" {
                disable-tunnel: w668 -> [w705 w715]
                disable-tunnel: w663 -> [w704 w712]
                disable-tunnel: [w705 w709] -> w667
                disable-tunnel: [w704 w707] -> w665
                frame Disabled {
                }
                frame Enabled {
                  n448 = local read "size limit"() -> (w711:i32)
                  n449 = local read "idxfront"() -> (w706:i32)
                  n450 = Array Subset(array=w715, index=0, length=w711) -> (w710:dbl[])
                  n451 = Array Subset(array=w712, index=0, length=w711) -> (w708:dbl[])
                  n452 = Array Subset(array=w710, index=w706) -> (w709:dbl[])  [unwired: 1 in]
                  n453 = Array Subset(array=w708, index=w706) -> (w707:dbl[])  [unwired: 1 in]
                }
              }
              n454 = Boolean To (0,1)(Boolean=w655) -> (0, 1=w656:i16[])
              n455 = Add Array Elements(numeric array=w693) -> (sum=w695:dbl)
              n456 = Add Array Elements(numeric array=w692) -> (sum=w694:dbl)
              n457 = To Long Integer(number=w656) -> (32bit integer=w657:i32[])
              n458 = Add Array Elements(numeric array=w657) -> (sum=w653:i32)
              n459 = local read "gap"() -> (w673:dbl)
              n460 = Max & Min(x=w653, y=1) -> (max(x,y)=w652:i32)  [unwired: 1 out]
              n461 = Divide(x=w680, y=w652) -> (x/y=w703:dbl)
              n462 = Divide(x=w695, y=w652) -> (x/y=w689:dbl)
              n463 = Divide(x=w694, y=w652) -> (x/y=w687:dbl)
              n464 = local read "af"() -> (w674:dbl)
              n465 = Divide(x=w673, y=w674) -> (x/y=w672:dbl)
              n466 = Multiply(x=w667, y=w672) -> (x*y=w661:dbl[])
              n467 = Add Array Elements(numeric array=w661) -> (sum=w679:dbl)
              n468 = Not Equal To 0?(x=w661) -> (x != 0?=w660:bool[])
              n469 = Polar To Re/Im(2:w665, 3:w661) -> (0:w669:dbl[], 1:w670:dbl[])
              n470 = Boolean To (0,1)(Boolean=w660) -> (0, 1=w659:i16[])
              n471 = Add Array Elements(numeric array=w670) -> (sum=w690:dbl)
              n472 = Add Array Elements(numeric array=w669) -> (sum=w691:dbl)
              n473 = To Long Integer(number=w659) -> (32bit integer=w658:i32[])
              n474 = Add Array Elements(numeric array=w658) -> (sum=w649:i32)
              n475 = Max & Min(x=w649, y=1) -> (max(x,y)=w648:i32)  [unwired: 1 out]
              n476 = Divide(x=w679, y=w648) -> (x/y=w702:dbl)
              n477 = Divide(x=w690, y=w648) -> (x/y=w688:dbl)
              n478 = Divide(x=w691, y=w648) -> (x/y=w671:dbl)
              n479 = Compound Arithmetic op=ADD(w689, w688) -> (w684:dbl)
              n480 = Compound Arithmetic op=ADD(w687, w671) -> (w681:dbl)
              n481 = Not A Number/Path/Refnum?(number/path/refnum=w684) -> (NaN/Path/Refnum?=w685:bool)
              n482 = Not A Number/Path/Refnum?(number/path/refnum=w681) -> (NaN/Path/Refnum?=w683:bool)
              n483 = Select(t=0.0, s=w685, f=w684) -> (s? t:f=w701:dbl)
              n484 = Select(t=0.0, s=w683, f=w681) -> (s? t:f=w700:dbl)
            }
            frame True {
            }
          }
          "rr_shift" <- w640
          "rf_shift" <- w639
          n485 = case shown="False" w616 {
            tunnel: [w809 _] -> w642
            tunnel: [w808 _] -> w641
            tunnel: [w807 _] -> w637
            tunnel: [w806 _] -> w635
            tunnel: w613 -> [w783 _]
            tunnel: w610 -> [w782 _]
            frame False {
              n486 = local read "h_path"() -> (w805:dbl[])
              n487 = local read "h_lf"() -> (w772:dbl[])
              n488 = local read "y_lf"() -> (w801:dbl[])
              n489 = local read "y_lr"() -> (w803:dbl[])
              n490 = local read "x_lf"() -> (w802:dbl[])
              n491 = local read "x_lr"() -> (w804:dbl[])
              n492 = for {
                tunnel: w783 -> [w847]
                tunnel: w782 -> [w846]
                tunnel: w805 -> [w834] mode=indexing
                tunnel: "d_safe front" -> [w848]
                tunnel: [w839] -> w771 mode=indexing
                tunnel: [w856] -> w775 mode=indexing
                tunnel: [w828] -> w757 mode=indexing
                tunnel: w804 -> [w845] mode=indexing
                tunnel: w803 -> [w844] mode=indexing
                tunnel: w802 -> [w843] mode=indexing
                tunnel: w801 -> [w842] mode=indexing
                tunnel: w772 -> [w824] mode=indexing
                tunnel: [w823] -> w770 mode=indexing
                tunnel: "d_safe" -> [w822]
                n493 = Subtract(x=w846, y=w842) -> (x-y=w850:dbl[])
                n494 = Subtract(x=w847, y=w843) -> (x-y=w849:dbl[])
                n495 = Subtract(x=w846, y=w844) -> (x-y=w837:dbl[])
                n496 = Subtract(x=w847, y=w845) -> (x-y=w838:dbl[])
                n497 = call "headingoperater.vi"("h1"=w824, "h2"=1.5707963267948966) -> ("h2-h1"=w827:dbl)  [unwired: 8 in, 1 out]
                n498 = call "headingoperater.vi"("h1"=w834, "h2"=1.5707963267948966) -> ("h2-h1"=w833:dbl)  [unwired: 8 in, 1 out]
                n499 = Square(x=w849) -> (x^2=w852:dbl[])
                n500 = Square(x=w850) -> (x^2=w851:dbl[])
                n501 = Square(x=w837) -> (x^2=w836:dbl[])
                n502 = Square(x=w838) -> (x^2=w835:dbl[])
                n503 = Add(x=w852, y=w851) -> (x+y=w853:dbl[])
                n504 = Add(x=w836, y=w835) -> (x+y=w859:dbl[])
                n505 = call "headingoperater.vi"("h1"=1.5707963267948966, "h2"=w827) -> ("h2-h1"=w823:dbl)  [unwired: 8 in, 1 out]
                n506 = call "headingoperater.vi"("h1"=1.5707963267948966, "h2"=w833) -> ("h2-h1"=w839:dbl)  [unwired: 8 in, 1 out]
                n507 = Square Root(x=w853) -> (sqrt(x)=w854:dbl[])
                n508 = Square Root(x=w859) -> (sqrt(x)=w858:dbl[])
                n509 = Array Max & Min(array=w854) -> (min value=w855:dbl)  [unwired: 3 out]
                n510 = Array Max & Min(array=w858) -> (min value=w857:dbl)  [unwired: 3 out]
                n511 = Subtract(x=w848, y=w855) -> (x-y=w829:dbl)
                n512 = Subtract(x=w822, y=w857) -> (x-y=w832:dbl)
                n513 = Max & Min(x=w829, y=0.0) -> (max(x,y)=w856:dbl)  [unwired: 1 out]
                n514 = Max & Min(x=w832, y=0.0) -> (max(x,y)=w828:dbl)  [unwired: 1 out]
              }
              n515 = Add Array Elements(numeric array=w757) -> (sum=w785:dbl)
              n516 = Not Equal To 0?(x=w757) -> (x != 0?=w761:bool[])
              n517 = Polar To Re/Im(2:w771, 3:w757) -> (0:w797:dbl[], 1:w798:dbl[])
              n518 = disable-structure shown="Enabled" {
                disable-tunnel: w775 -> [w810 w819]
                disable-tunnel: [w811 w813] -> w773
                disable-tunnel: w770 -> [w811 w818]
                disable-tunnel: [w810 w815] -> w774
                frame Disabled {
                }
                frame Enabled {
                  n519 = local read "size limit"() -> (w817:i32)
                  n520 = local read "idxfront"() -> (w812:i32)
                  n521 = Array Subset(array=w819, index=0, length=w817) -> (w816:dbl[])
                  n522 = Array Subset(array=w818, index=0, length=w817) -> (w814:dbl[])
                  n523 = Array Subset(array=w816, index=w812) -> (w815:dbl[])  [unwired: 1 in]
                  n524 = Array Subset(array=w814, index=w812) -> (w813:dbl[])  [unwired: 1 in]
                }
              }
              n525 = Boolean To (0,1)(Boolean=w761) -> (0, 1=w760:i16[])
              n526 = Add Array Elements(numeric array=w798) -> (sum=w800:dbl)
              n527 = Add Array Elements(numeric array=w797) -> (sum=w799:dbl)
              n528 = To Long Integer(number=w760) -> (32bit integer=w759:i32[])
              n529 = Add Array Elements(numeric array=w759) -> (sum=w758:i32)
              n530 = local read "gap"() -> (w781:dbl)
              n531 = Max & Min(x=w758, y=1) -> (max(x,y)=w756:i32)  [unwired: 1 out]
              n532 = Divide(x=w785, y=w756) -> (x/y=w809:dbl)
              n533 = Divide(x=w800, y=w756) -> (x/y=w794:dbl)
              n534 = Divide(x=w799, y=w756) -> (x/y=w792:dbl)
              n535 = local read "af"() -> (w780:dbl)
              n536 = Divide(x=w781, y=w780) -> (x/y=w778:dbl)
              n537 = Multiply(x=w774, y=w778) -> (x*y=w763:dbl[])
              n538 = Add Array Elements(numeric array=w763) -> (sum=w784:dbl)
              n539 = Not Equal To 0?(x=w763) -> (x != 0?=w767:bool[])
              n540 = Polar To Re/Im(2:w773, 3:w763) -> (0:w776:dbl[], 1:w777:dbl[])
              n541 = Boolean To (0,1)(Boolean=w767) -> (0, 1=w766:i16[])
              n542 = Add Array Elements(numeric array=w777) -> (sum=w795:dbl)
              n543 = Add Array Elements(numeric array=w776) -> (sum=w796:dbl)
              n544 = To Long Integer(number=w766) -> (32bit integer=w765:i32[])
              n545 = Add Array Elements(numeric array=w765) -> (sum=w764:i32)
              n546 = Max & Min(x=w764, y=1) -> (max(x,y)=w762:i32)  [unwired: 1 out]
              n547 = Divide(x=w784, y=w762) -> (x/y=w808:dbl)
              n548 = Divide(x=w795, y=w762) -> (x/y=w793:dbl)
              n549 = Divide(x=w796, y=w762) -> (x/y=w779:dbl)
              n550 = Compound Arithmetic op=ADD(w794, w793) -> (w789:dbl)
              n551 = Compound Arithmetic op=ADD(w792, w779) -> (w786:dbl)
              n552 = Not A Number/Path/Refnum?(number/path/refnum=w789) -> (NaN/Path/Refnum?=w790:bool)
              n553 = Not A Number/Path/Refnum?(number/path/refnum=w786) -> (NaN/Path/Refnum?=w788:bool)
              n554 = Select(t=0.0, s=w790, f=w789) -> (s? t:f=w807:dbl)
              n555 = Select(t=0.0, s=w788, f=w786) -> (s? t:f=w806:dbl)
            }
            frame True {
            }
          }
          "lr_shift" <- w642
          "lf_shift" <- w641
          n556 = Add(x=w638, y=w637) -> (x+y=w624:dbl)
          n557 = Add(x=w636, y=w635) -> (x+y=w618:dbl)
          n558 = Absolute Value(x=w624) -> (abs(x)=w628:dbl)
          n559 = Absolute Value(x=w618) -> (abs(x)=w619:dbl)
          n560 = Less?(x=w628, y=0.0001) -> (x < y?=w626:bool)
          n561 = Less?(x=w619, y=0.0001) -> (x < y?=w621:bool)
          n562 = Select(t=0.0, s=w626, f=w624) -> (s? t:f=w623:dbl)
          "x_shift" <- w623
          n563 = Select(t=0.0, s=w621, f=w618) -> (s? t:f=w617:dbl)
          "y_shift" <- w617
          n564 = Absolute Value(x="x limit") -> (abs(x)=w630:dbl)
          n565 = Absolute Value(x="y limit") -> (abs(x)=w597:dbl)
          n566 = Multiply(x=w623, y="x_gain") -> (x*y=w632:dbl)
          n567 = Negate(x=w630) -> (-x=w629:dbl)
          n568 = Multiply(x="y_gain", y=w617) -> (x*y=w601:dbl)
          n569 = Negate(x=w597) -> (-x=w599:dbl)
          n570 = In Range and Coerce(upper limit=w630, x=w632, lower limit=w629) -> (coerced(x)=w595:dbl)  [unwired: 1 out]
          n571 = In Range and Coerce(upper limit=w597, x=w601, lower limit=w599) -> (coerced(x)=w600:dbl)  [unwired: 1 out]
          n572 = disable-structure shown="Disabled" {
            disable-tunnel: [w643 _] -> w596
            disable-tunnel: w595 -> [w643 _]
            frame Disabled {
            }
            frame Enabled {
            }
          }
          n573 = global write "G_SEN.vi" "laser y shift"(w600) -> ()
          n574 = global write "G_SEN.vi" "laser x shift"(w596) -> ()
        }
        frame #7 {
          n575 = local read "R0"() -> (w909:dbl)
          n576 = local read "r"() -> (w908:dbl[])
          n577 = local read "rout"() -> (w899:dbl[])
          n578 = local read "rin"() -> (w905:dbl[])
          n579 = Reciprocal(x=w908) -> (1/x=w907:dbl[])
          n580 = Reciprocal(x=w909) -> (1/x=w906:dbl)
          n581 = Reciprocal(x=w899) -> (1/x=w900:dbl[])
          n582 = Threshold 1D Array(2:w906, 3:w907) -> (0:w898:dbl)  [unwired: 1 in]
          n583 = Reciprocal(x=w905) -> (1/x=w904:dbl[])
          n584 = Interpolate 1D Array(1:w898, 2:w904) -> (0:w903:dbl)
          n585 = Interpolate 1D Array(1:w898, 2:w900) -> (0:w901:dbl)
          n586 = local read "size limit"() -> (w863:i32)
          n587 = local read "R0"() -> (w896:dbl)
          n588 = Reciprocal(x=w903) -> (1/x=w902:dbl)
          n589 = Reciprocal(x=w901) -> (1/x=w897:dbl)
          n590 = local read "size limit"() -> (w869:i32)
          n591 = local read "y_lf"() -> (w879:dbl[])
          n592 = local read "y_rf"() -> (w877:dbl[])
          n593 = Absolute Value(x=w896) -> (abs(x)=w951:dbl)
          n594 = Absolute Value(x=w902) -> (abs(x)=w946:dbl)
          n595 = Absolute Value(x=w897) -> (abs(x)=w941:dbl)
          n596 = local read "idxfront"() -> (w860:i32)
          n597 = local read "theta"() -> (w952:dbl[])
          n598 = local read "theta"() -> (w945:dbl[])
          n599 = local read "theta"() -> (w942:dbl[])
          n600 = Array Subset(array=w879, index=0, length=w863) -> (w862:dbl[])
          n601 = Array Subset(array=w877, index=0, length=w863) -> (w861:dbl[])
          n602 = local read "x_rf"() -> (w872:dbl[])
          n603 = local read "x_lf"() -> (w875:dbl[])
          n604 = local read "idxfront"() -> (w868:i32)
          n605 = local read "y_path"() -> (w921:dbl[])
          n606 = local read "y_shift"() -> (w886:dbl)
          n607 = local read "y_path"() -> (w887:dbl[])
          n608 = Array Subset(array=w875, index=0, length=w869) -> (w867:dbl[])
          n609 = Array Subset(array=w872, index=0, length=w869) -> (w866:dbl[])
          n610 = Array Subset(array=w862, index=w860) -> (w878:dbl[])  [unwired: 1 in]
          n611 = Array Subset(array=w861, index=w860) -> (w876:dbl[])  [unwired: 1 in]
          n612 = Polar To Re/Im(2:w952, 3:w951) -> (0:w948:dbl[], 1:w950:dbl[])
          n613 = Polar To Re/Im(2:w945, 3:w946) -> (0:w943:dbl[], 1:w947:dbl[])
          n614 = Polar To Re/Im(2:w942, 3:w941) -> (0:w938:dbl[], 1:w940:dbl[])
          n615 = local read "y_lr"() -> (w920:dbl[])
          n616 = local read "y_rr"() -> (w916:dbl[])
          n617 = local read "x_path"() -> (w931:dbl[])
          n618 = local read "x_shift"() -> (w890:dbl)
          n619 = local read "x_path"() -> (w891:dbl[])
          n620 = local read "y_car"() -> (w913:dbl[])
          n621 = Add(x=w896, y=w950) -> (x+y=w949:dbl[])
          n622 = Add(x=w896, y=w947) -> (x+y=w944:dbl[])
          n623 = Add(x=w896, y=w940) -> (x+y=w939:dbl[])
          n624 = Add(x=w886, y=w887) -> (x+y=w885:dbl[])
          n625 = Array Subset(array=w867, index=w868) -> (w874:dbl[])  [unwired: 1 in]
          n626 = Array Subset(array=w866, index=w868) -> (w873:dbl[])  [unwired: 1 in]
          n627 = local read "x_lr"() -> (w923:dbl[])
          n628 = local read "x_rr"() -> (w919:dbl[])
          n629 = call "Convert to Dynamic Data8"("Array"=w948) -> ("Dynamic Data Type"=w934:dynamicdata)  [unwired: 3 in]
          n630 = call "Convert to Dynamic Data10"("Array"=w943) -> ("Dynamic Data Type"=w933:dynamicdata)  [unwired: 3 in]
          n631 = call "Convert to Dynamic Data12"("Array"=w938) -> ("Dynamic Data Type"=w932:dynamicdata)  [unwired: 3 in]
          n632 = call "Convert to Dynamic Data15"("Array"=w921) -> ("Dynamic Data Type"=w926:dynamicdata)  [unwired: 3 in]
          n633 = call "Convert to Dynamic Data16"("Array"=w878) -> ("Dynamic Data Type"=w927:dynamicdata)  [unwired: 3 in]
          n634 = call "Convert to Dynamic Data17"("Array"=w920) -> ("Dynamic Data Type"=w924:dynamicdata)  [unwired: 3 in]
          n635 = call "Convert to Dynamic Data21"("Array"=w876) -> ("Dynamic Data Type"=w915:dynamicdata)  [unwired: 3 in]
          n636 = call "Convert to Dynamic Data22"("Array"=w916) -> ("Dynamic Data Type"=w914:dynamicdata)  [unwired: 3 in]
          n637 = local read "yr"() -> (w880:dbl[])
          n638 = local read "yl"() -> (w882:dbl[])
          n639 = local read "y"() -> (w895:dbl[])
          n640 = local read "x_car"() -> (w911:dbl[])
          n641 = Merge Signals(w926, w927, w924, w915, w914) -> (w925:dynamicdata)
          n642 = Merge Signals(w934, w933, w932) -> (w892:dynamicdata)
          n643 = Add(x=w890, y=w891) -> (x+y=w889:dbl[])
          n644 = call "Convert to Dynamic Data7"("Array"=w949) -> ("Dynamic Data Type"=w937:dynamicdata)  [unwired: 3 in]
          n645 = call "Convert to Dynamic Data9"("Array"=w944) -> ("Dynamic Data Type"=w936:dynamicdata)  [unwired: 3 in]
          n646 = call "Convert to Dynamic Data11"("Array"=w939) -> ("Dynamic Data Type"=w935:dynamicdata)  [unwired: 3 in]
          n647 = call "Convert to Dynamic Data13"("Array"=w931) -> ("Dynamic Data Type"=w930:dynamicdata)  [unwired: 3 in]
          n648 = call "Convert to Dynamic Data14"("Array"=w874) -> ("Dynamic Data Type"=w929:dynamicdata)  [unwired: 3 in]
          n649 = call "Convert to Dynamic Data18"("Array"=w923) -> ("Dynamic Data Type"=w922:dynamicdata)  [unwired: 3 in]
          n650 = call "Convert to Dynamic Data19"("Array"=w873) -> ("Dynamic Data Type"=w918:dynamicdata)  [unwired: 3 in]
          n651 = call "Convert to Dynamic Data20"("Array"=w919) -> ("Dynamic Data Type"=w917:dynamicdata)  [unwired: 3 in]
          n652 = call "Convert to Dynamic Data23"("Array"=w913) -> ("Dynamic Data Type"=w912:dynamicdata)  [unwired: 3 in]
          n653 = call "Convert to Dynamic Data26"("Array"=w885) -> ("Dynamic Data Type"=w884:dynamicdata)  [unwired: 3 in]
          n654 = call "Convert to Dynamic Data2"("Array"=w895) -> ("Dynamic Data Type"=w961:dynamicdata)  [unwired: 3 in]
          n655 = call "Convert to Dynamic Data6"("Array"=w880) -> ("Dynamic Data Type"=w953:dynamicdata)  [unwired: 3 in]
          n656 = call "Convert to Dynamic Data4"("Array"=w882) -> ("Dynamic Data Type"=w955:dynamicdata)  [unwired: 3 in]
          n657 = local read "xl"() -> (w883:dbl[])
          n658 = local read "xr"() -> (w881:dbl[])
          n659 = local read "x"() -> (w894:dbl[])
          n660 = Merge Signals(w937, w936, w935) -> (w893:dynamicdata)
          n661 = Merge Signals(w930, w929, w922, w918, w917) -> (w928:dynamicdata)
          n662 = call "Convert to Dynamic Data24"("Array"=w911) -> ("Dynamic Data Type"=w910:dynamicdata)  [unwired: 3 in]
          n663 = call "Convert to Dynamic Data25"("Array"=w889) -> ("Dynamic Data Type"=w888:dynamicdata)  [unwired: 3 in]
          n664 = Merge Signals(w961, w955, w953, w892, w925, w912, w884) -> (w956:dynamicdata)
          n665 = call "Convert to Dynamic Data3"("Array"=w883) -> ("Dynamic Data Type"=w957:dynamicdata)  [unwired: 3 in]
          n666 = call "Convert to Dynamic Data"("Array"=w894) -> ("Dynamic Data Type"=w960:dynamicdata)  [unwired: 3 in]
          n667 = call "Convert to Dynamic Data5"("Array"=w881) -> ("Dynamic Data Type"=w954:dynamicdata)  [unwired: 3 in]
          n668 = Merge Signals(w960, w957, w954, w893, w928, w910, w888) -> (w958:dynamicdata)
          n669 = call "Build XY Graph"("Y Input"=w956, "X Input"=w958) -> ("XY Graph"=→"XY Graph":cluster{"X":dbl[], "Y":dbl[]}[])  [unwired: 8 in, 1 out]
        }
      }
    }
  }
